vi "PulseGenPan.vi"(8 "error in (no error)":errorcluster caption="entrée d'erreur (pas d'erreur)", 11 "DAQ6363.lvclass":refnum<class "DAQ6363.lvclass">) -> (0 "error out":errorcluster caption="sortie d'erreur", 3 "DAQ6363.lvclass Out":refnum<class "DAQ6363.lvclass">)   [LabVIEW 2019, in "DAQ6363.lvclass"]
uses:
  DAQ6363.lvclass
  C:/Programmes Labview/LabscanV1A/DevicesClass/BaseDevice/BaseDevice.lvclass
  BaseDevice/ClassQueueMess.ctl
  DAQ6363_Func.ctl
  DAQ6363.lvclass/DAQ6363.ctl
  BaseDevice/BaseDevice.lvclass/BaseDevice.ctl
  BaseDevice/Accessor/SetShowInstrNm.vi
  BaseDevice/Accessor/GetClassEvent.vi
  <vilib>/DAQmx/create/channels.llb/DAQmx Create Channel (CI-Count Edges).vi
  <vilib>/DAQmx/create/channels.llb/DAQmx Create Channel (CO-Pulse Generation-Time).vi
  <vilib>/DAQmx/configure/timing.llb/DAQmx Timing (Implicit).vi
  <vilib>/DAQmx/configure/trigger.llb/DAQmx Start Trigger (Digital Edge).vi
  <resource>/objmgr/daqmx.rc
panel:
  in  "MWP":i32=1
  out "APD2GateTask":refnum<k21> caption="tâche en sortie"
  out "Det2CntTask":refnum<k21> caption="tâche en sortie"
  in  "Mw initial delay(s) 2":dbl caption="retard initial" format="%.6f"
  out "LaserLowTime":dbl
  in  "Mw initial delay(s)":dbl caption="retard initial" format="%.6f"
  out "ControlsNames":string[](array[string])
  out "DetCntTask":refnum<k21> caption="tâche en sortie"
  out "APDTask":refnum<k21> caption="tâche en sortie"
  out "MWTask":refnum<k21> caption="tâche en sortie"
  out "LaserTask":refnum<k21> caption="tâche en sortie"
  out "ReadCnts":bool
  in  "DAQ6363 Tabs":enum32{"Main", "Pulsed ODMR", "Advanced"}(tab)
  in  "APD Gate":bool
  in  "Pulse Function":T1(ring)
  in  "Channel 1":bool
  in  "Channel 2":bool
  in  "Rate Graph":bool caption="Rate\nGraph"
  in  "ReadCont":bool caption="Read\nCont."
  out "ReadCounts 2":u32=100 caption="Counts Ch2" min=1 max=100000 step=1
  out "CountsPerSec 2":dbl=100.0 caption="Counts/s Ch2" min=1.0 max=100000.0 step=1.0
  in  "LS_APD_Dl_us 2":dbl=0.02 caption="Laser-APD2\nDelay (us)" min=0.01 max=1000000000.0 step=0.01
  out "ReadCounts":u32=100 caption="Counts Ch1" min=1 max=100000 step=1
  in  "AquireODMR":bool caption="MiseAJour"
  in  "Stop Acq":bool
  in  "APDTime_us":dbl=2.0 caption="APD Gate\nTime (us)" min=0.01 max=1000000000.0 step=0.01
  in  "LS_APD_Dl_us":dbl=0.02 caption="Laser-APD\nDelay (us)" min=0.01 max=1000000000.0 step=0.01
  in  "LS_MW_Dl_us":dbl=0.15 caption="Laser-MW\nDelay (us)" min=0.01 max=1000000000.0 step=0.01
  in  "MW_LS_Dl_us":dbl=0.1 caption="MW-Laser\nDelay (us)" min=0.01 max=1000000000.0 step=0.01
  in  "MWTime_us":dbl=4.0 caption="Microwave\nOn Time (us)" min=0.01 max=1000000000.0 step=0.01
  in  "PulseCount":i32=30000 caption="Avg. Pulses" min=1 step=1
  in  "LaserTime_us":dbl=10.0 caption="Laser On\nTime (us)" min=0.01 max=1000000000.0 step=0.01
  out "AcqTime":dbl caption="AcqTime(s)" format="%<%M:%S%3u>t"
  out "CountsPerSec":dbl=100.0 caption="Counts/s Ch1" min=1.0 max=100000.0 step=1.0
  out "Period(us)":dbl
  in  "DetInput2":tag="/Dev1/PFI8" caption="Detection Input 2"
  in  "DetCntr 2":tag="Dev1/ctr3" caption="Detection Counter 2"
  in  "APDOutput 2":tag="/Dev1/PFI11" caption="APD Gate In/Out 2"
  in  "APDGateCntr2":tag="Dev1/ctr2" caption="APD Gate Counter 2"
  in  "DetInput":tag="/Dev1/PFI13" caption="Detection Input"
  in  "DetCntr":tag="Dev1/ctr0" caption="Detection Counter"
  in  "APDCntr":tag="Dev1/ctr1" caption="APD Gate Counter"
  in  "APDOutput":tag="/Dev1/PFI10" caption="APD Gate In/Out"
  in  "MWCntr":tag="Dev1/ctr2" caption="Microwave Counter"
  in  "LaserCntr":tag="Dev1/ctr1" caption="Laser Counter"
  in  "Laser In/Out":tag="/Dev1/PFI9" caption="LaserTrig In/Out"
  in  "MW In/Out":tag="/Dev1/PFI12" caption="Microwave In/Out"
  in  "APDGateEdge":i32(ring)=10280 items=["Montant"=10280, "Descendant"=10171]
  in  "MainProgQ":refnum<queue>
  in  "MainProgQEvent":refnum<user-event>
  in  "Acq":bool
  in  "Stop":bool
  out "Init Program":bool
  # "DAQ6363 Pulse Gen"
  # "this MUST labeled with class name"
  # "this MUST be present and labeled \"Stop\" and \"Acq\""
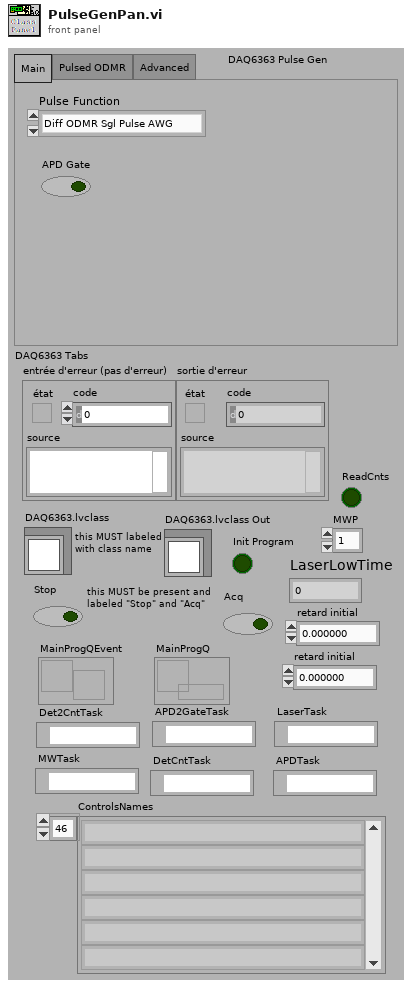
[diagram p1: front panel]
types:
  T1 = enum16{"Diff ODMR Sgl Pulse AWG", "Pulsed ODMR AWG", "Diff Pulsed ODMR AWG", "Pulsed ODMR", "Diff Pulsed ODMR", "Ramsey", "Rabi", "Gated Pulse Count", "None"}
  T2 = typedef "DAQ6363.lvclass/DAQ6363_Func.ctl" = enum16{"CountPulse (Cnt)", "Rabi (Tau)", "MWtoLaserDelay (us)", "APDGate (us)", "PulsedODMR (Pulses)", "PulsedODMR_AWG (Pulses)", "DiffODMRSglPulseAWG (Pulses)", "DiffPulsedODMR_AWG (Pulses)", "GatedPulseCount (Pulses)", "DiffPulsedODMR (Pulses)"}
  T3 = typedef "ClassQueueMess.ctl" = u16
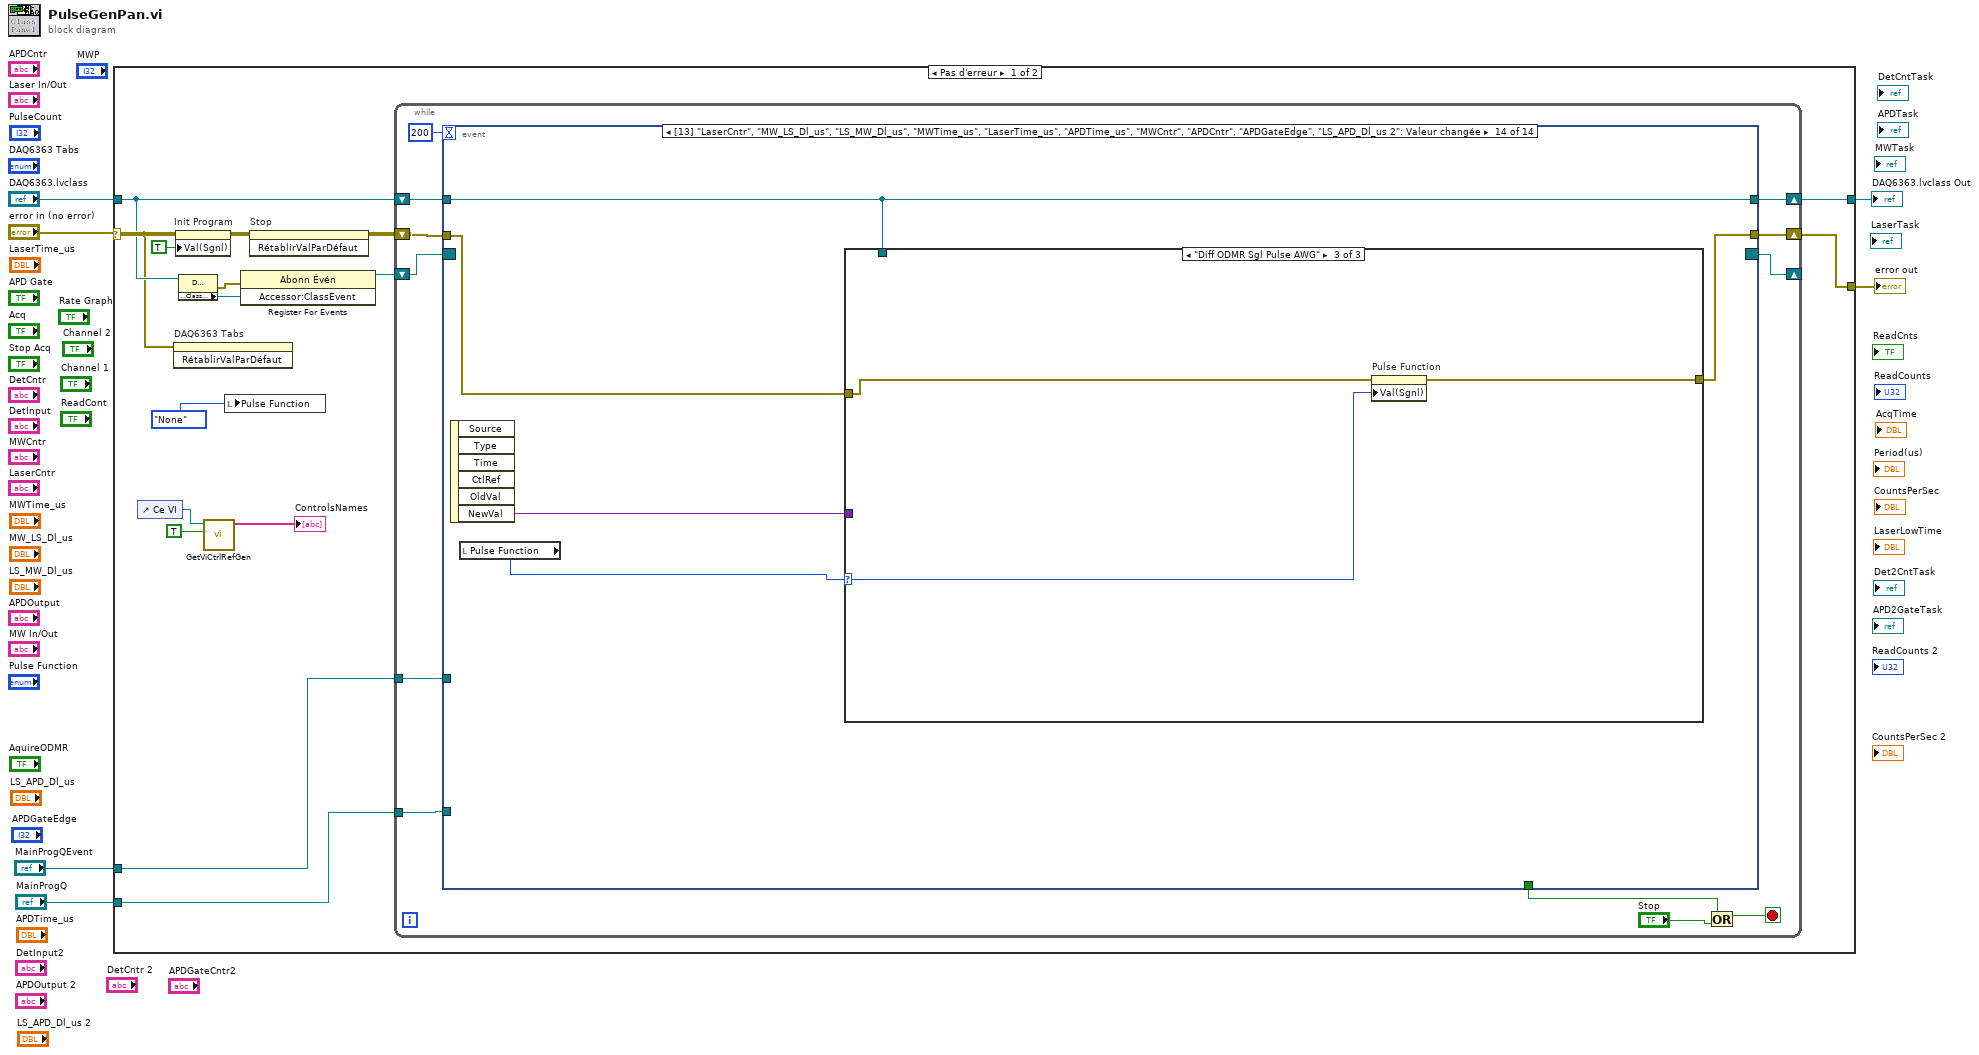
[diagram p0: block diagram]
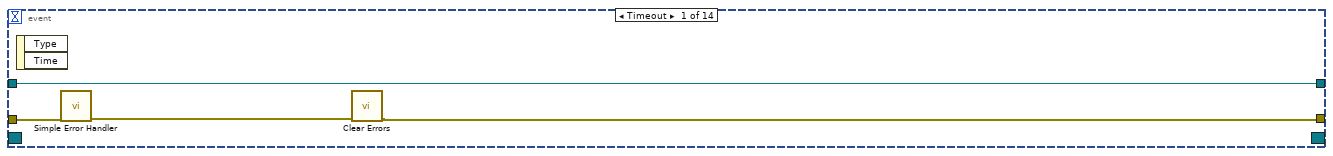
[diagram p2: hidden frame]
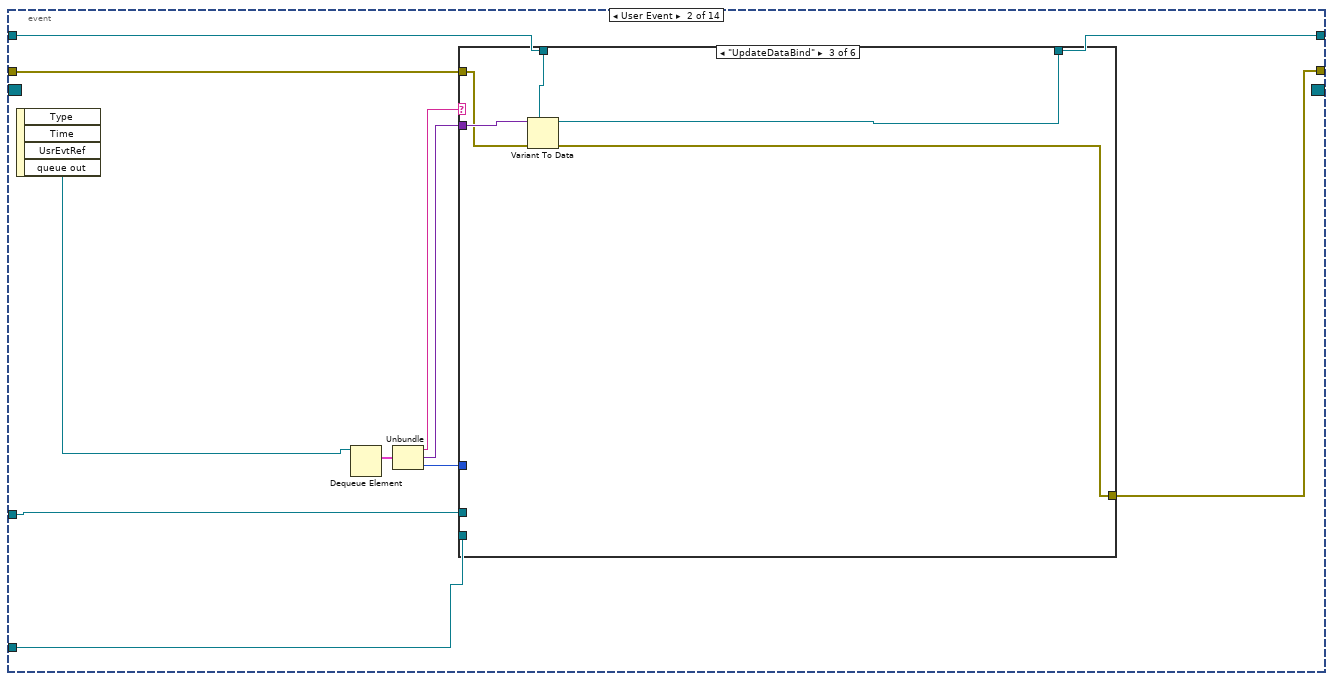
[diagram p3: hidden frame]
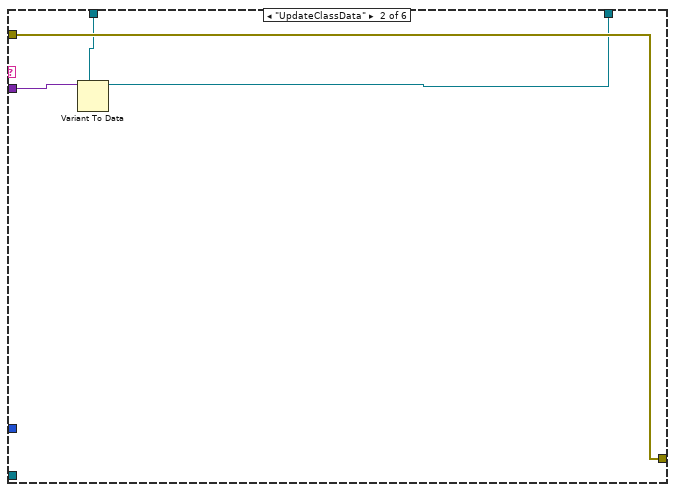
[diagram p5: hidden frame]
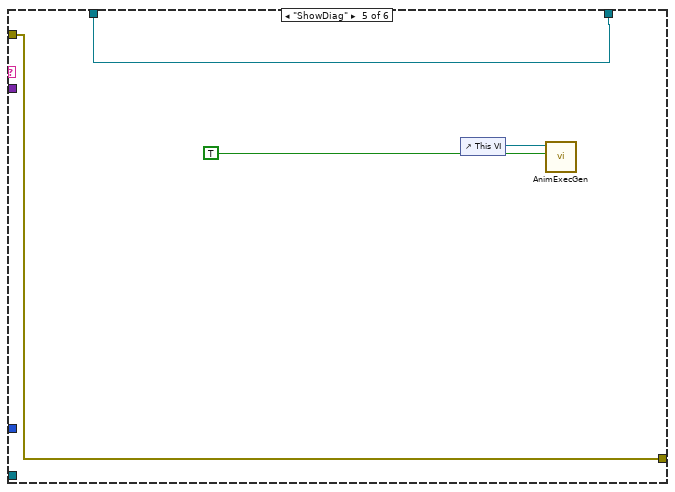
[diagram p7: hidden frame]
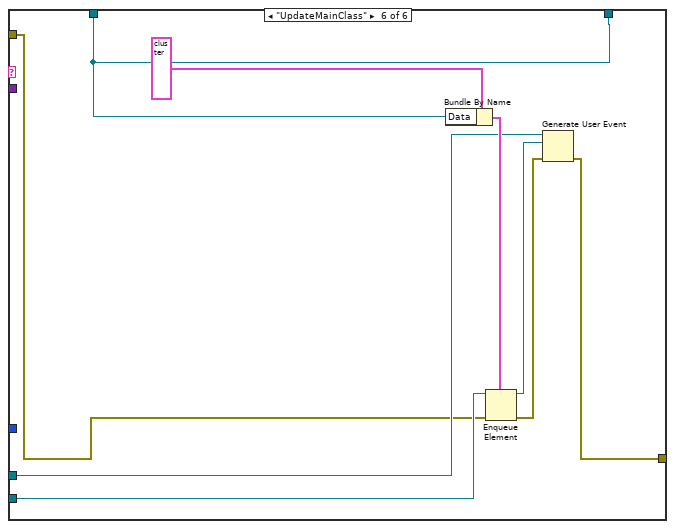
[diagram p8: hidden frame]
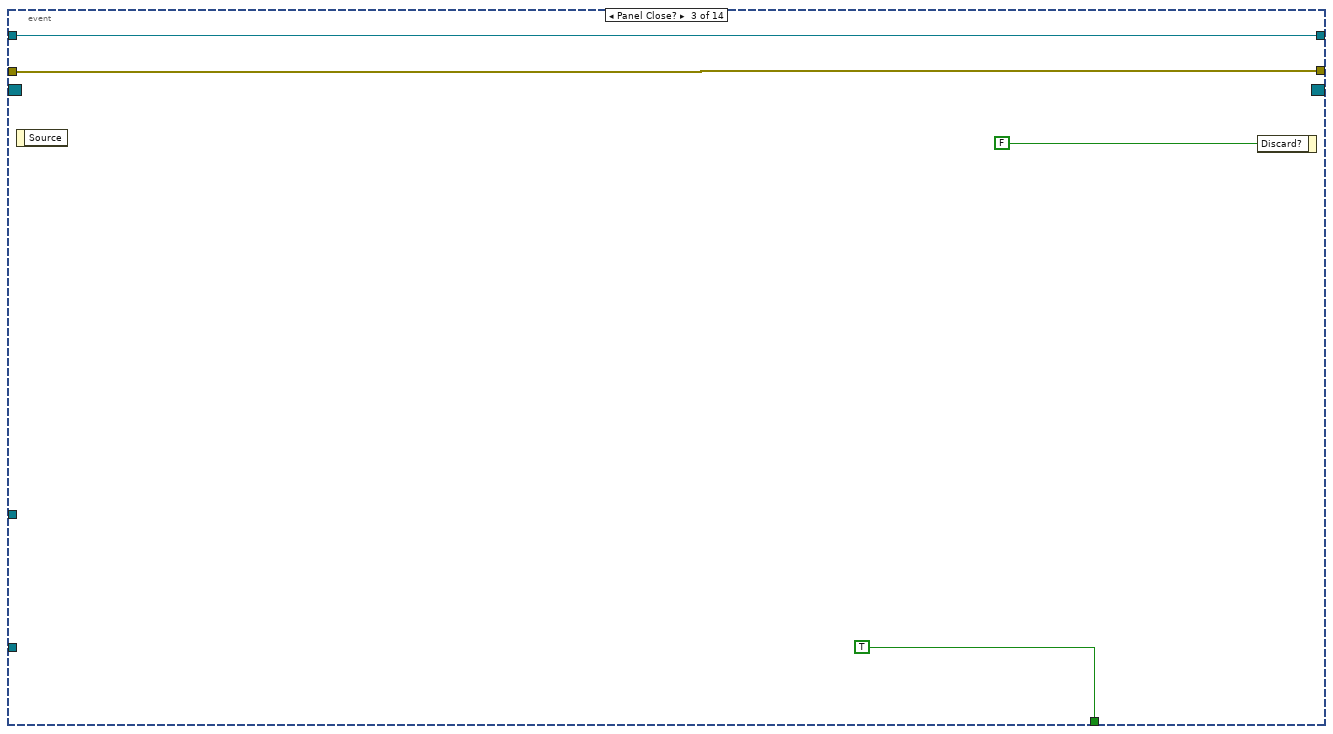
[diagram p9: hidden frame]
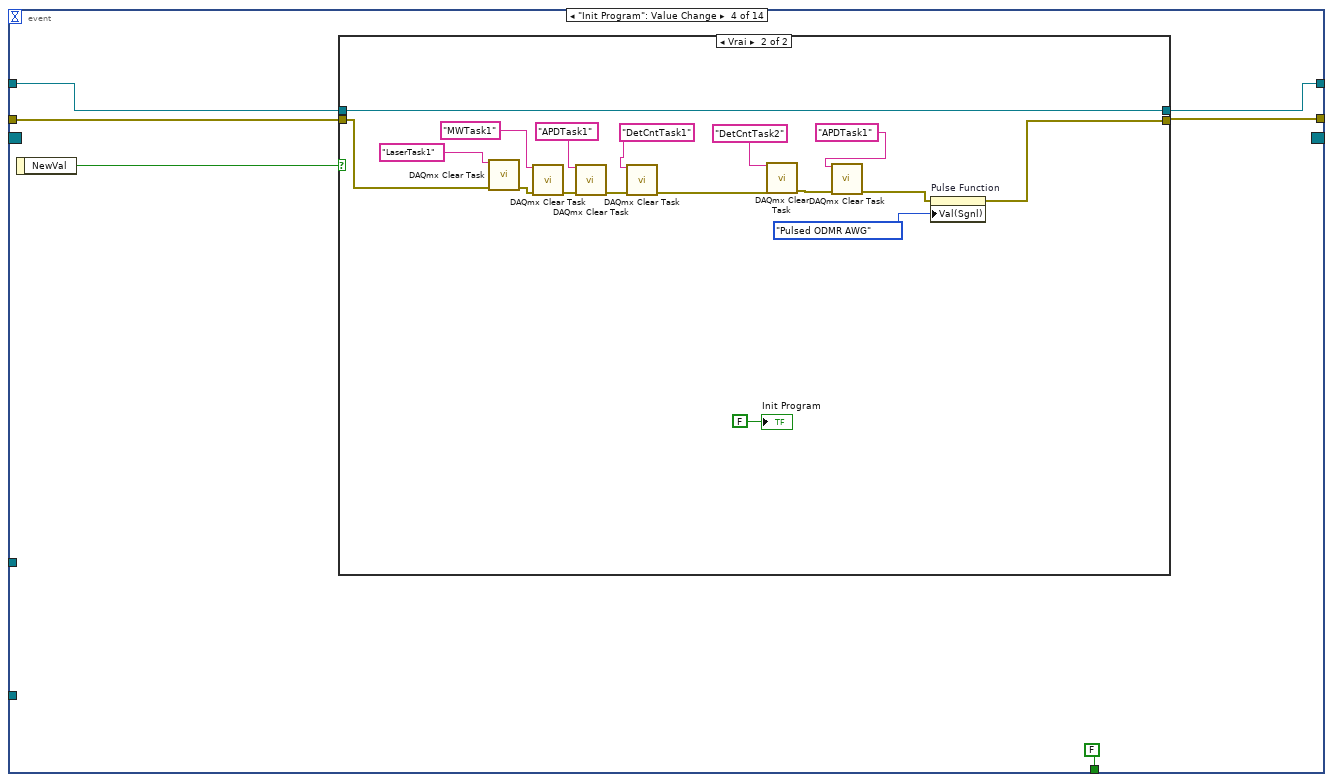
[diagram p10: hidden frame]
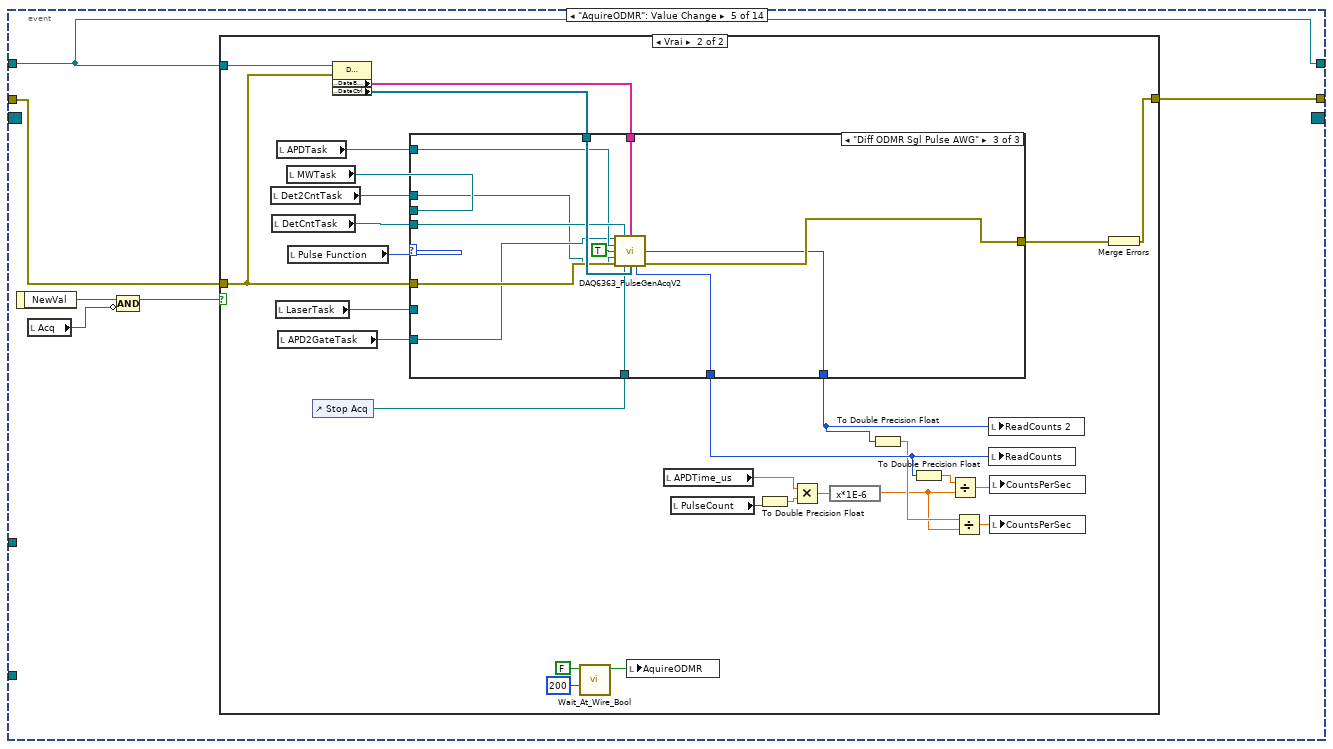
[diagram p12: hidden frame]
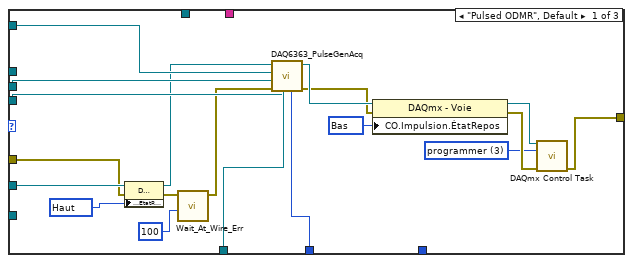
[diagram p14: hidden frame]
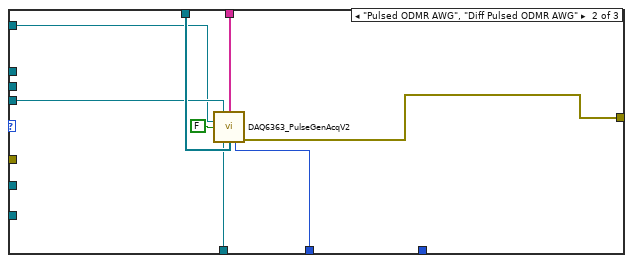
[diagram p15: hidden frame]
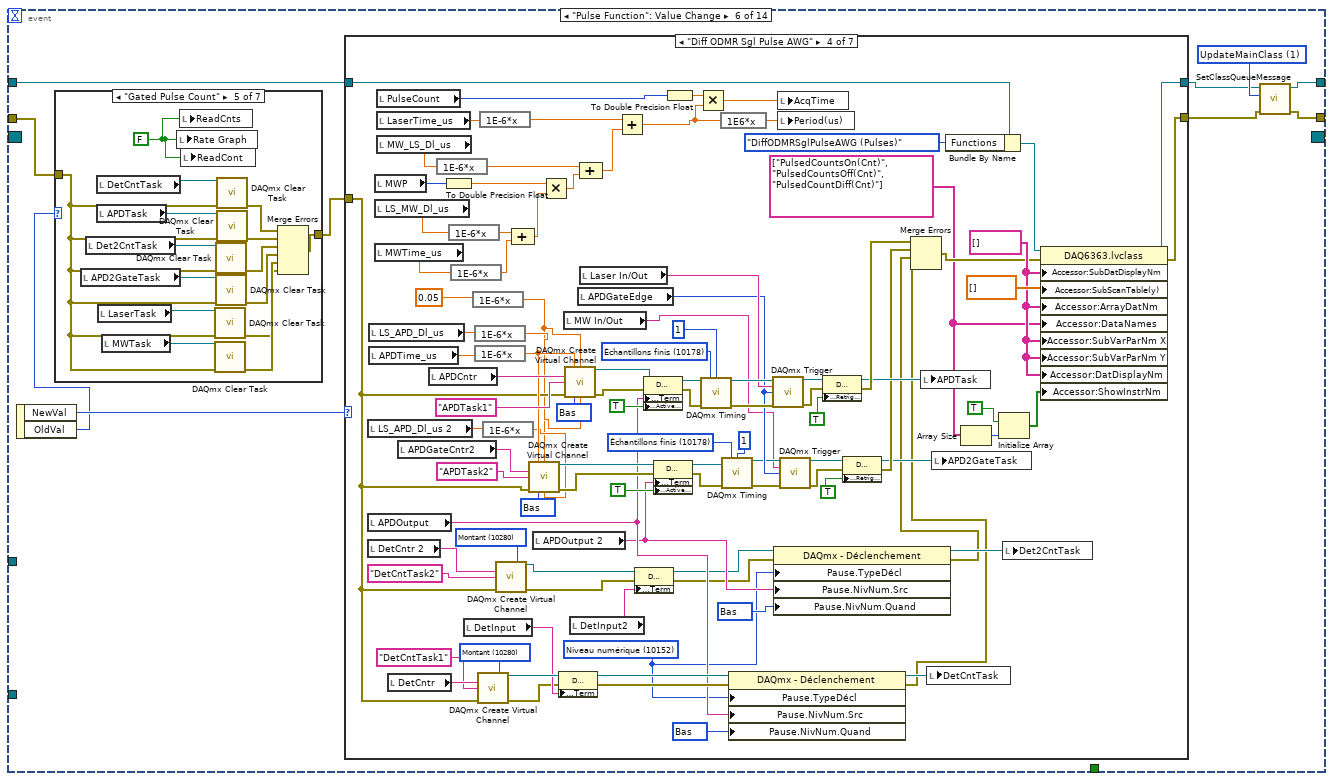
[diagram p16: hidden frame]
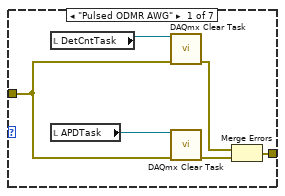
[diagram p17: hidden frame]
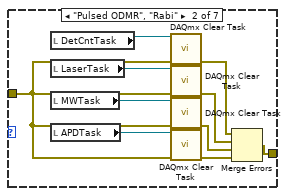
[diagram p18: hidden frame]
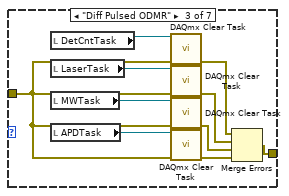
[diagram p19: hidden frame]
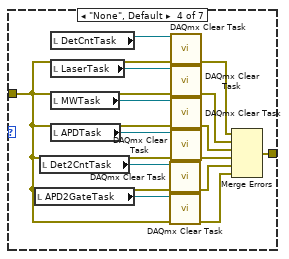
[diagram p20: hidden frame]
diagram:
  n1 = case shown="Pas d'erreur" "error in (no error)" {
    selector: "error in (no error)" -> [w11 w908]
    tunnel: [w22 w908] -> w5
    tunnel: "DAQ6363.lvclass" -> [w15 w907]
    tunnel: [w20 w907] -> w3
    tunnel: "MainProgQEvent" -> [w13 _]
    tunnel: "MainProgQ" -> [w12 _]
    frame No Error {
      n2 = control-ref of="Ce VI"() -> (w9:refnum<vi>)
      n3 = invoke on="DAQ6363 Tabs" class="Onglet (strict)" method="RétablirValParDéfaut"(error in=w11) -> ()  [unwired: 2 in, 3 out]
      n4 = property on="Init Program" class="Bool (strict)"(error in=w11, "Val(Sgnl)"=TRUE ("Valeur (Signalisation)")) -> (error out=w19:errorcluster)  [unwired: 1 in, 1 out]
      n5 = property class="DAQ6363.lvclass"(reference=w15) -> (error out=w17:errorcluster, "Accessor:ClassEvent"=w16:refnum<user-event>)  [unwired: 1 in, 1 out]
      n6 = call <userlib>:"GetViCtrlRefGen.vi"("InclTabCTrl"=TRUE, "VIRef"=w9) -> ("ControlsNames"=→"ControlsNames":string[])  [unwired: 7 in, 2 out]
      n7 = local write "Pulse Function"(T1."None" ("Pulse Function")) -> ()
      n8 = register-events(error in=w17, w16) -> (reference out=w14:refnum<event-registration>)  [unwired: 1 in, 1 out]
      n9 = invoke on="Stop" class="Bool (strict)" method="RétablirValParDéfaut"(error in=w19) -> (error out=w18:errorcluster)  [unwired: 2 in, 2 out]
      n10 = while {
        shift-right: [w32] -> w22
        shift-left: w18 -> [w33]
        shift-right: [w30] -> w20
        shift-left: w15 -> [w31]
        shift-right: [w26] -> _
        shift-left: w14 -> [w27]
        tunnel: w13 -> [w25]
        tunnel: w12 -> [w24]
        stop <- w29 stop-if-true
        n11 = event shown="[13] \"LaserCntr\", \"MW_LS_Dl_us\", \"LS_MW_Dl_us\", \"MWTime_us\", \"LaserTime_us\", \"APDTime_us\", \"MWCntr\", \"APDCntr\", \"APDGateEdge\", \"LS_APD_Dl_us 2\": Valeur changée" {
          selector: w27 -> [_ _ _ _ _ _ _ _ _ _ _ _ _ _]
          dyn-events: [_ _ _ _ _ _ _ _ _ _ _ _ _ _] -> w26
          timeout: 200 -> [_ _ _ _ _ _ _ _ _ _ _ _ _ _]
          tunnel: w33 -> [w38 w48 w77 w84 w109 w180 w722 w781 w827 w843 w867 w877 w887 w897]
          tunnel: [w35 w42 w77 w83 w108 w186 w719 w778 w829 w842 w866 w876 w886 w896] -> w32
          tunnel: w31 -> [w36 w49 w76 w81 w105 w188 w723 w782 w830 w844 w868 w878 w888 w898]
          tunnel: [w36 w41 w76 w80 w105 w184 w717 w776 w830 w844 w868 w878 w888 w898] -> w30
          tunnel: w25 -> [_ w40 _ _ _ _ _ _ _ _ _ _ _ _]
          tunnel: w24 -> [_ w39 _ _ _ _ _ _ _ _ _ _ _ _]
          tunnel: [_ _ TRUE FALSE _ _ _ _ _ _ _ _ _ _] -> w23
          event Timeout {
            n12 = event-data() -> ()  [unwired: 1 in, 2 out]
            n13 = call <vilib>:"Simple Error Handler.vi"("error in (no error)"=w38) -> ("error out"=w37:errorcluster)  [unwired: 4 in, 4 out]
            n14 = call <vilib>:"Clear Errors.vi"("error in (no error)"=w37) -> ("error out"=w35:errorcluster)  [unwired: 5 in, 1 out]
          }
          event User Event {
            n15 = event-data() -> ("queue out"=w46:refnum<queue>)  [unwired: 1 in, 3 out]
            n16 = Dequeue Element(queue=w46) -> (element=w47:cluster{"Message":string, "Data":variant, i32})  [unwired: 2 in, 3 out]
            n17 = Unbundle(w47) -> ("Message"=w45:string, "Data"=w44:variant, w43:i32)
            n18 = case shown="\"UpdateDataBind\"" w45 {
              tunnel: w48 -> [w51 w55 w57 w61 w65 w68]
              tunnel: w44 -> [_ w54 w60 _ _ _]
              tunnel: w49 -> [w50 w53 w59 w62 w66 w71]
              tunnel: [w50 w52 w58 w62 w66 w71] -> w41
              tunnel: [w51 w55 w56 w61 w65 w67] -> w42
              tunnel: w43 -> [_ _ _ _ _ _]
              tunnel: w40 -> [_ _ _ _ _ w70]
              tunnel: w39 -> [_ _ _ _ _ w69]
              frame Default {
              }
              frame "UpdateClassData" {
                n19 = Variant To Data(type=w53, Variant=w54) -> (data=w52:refnum<class "DAQ6363.lvclass">)  [unwired: 1 in, 1 out]
              }
              frame "UpdateDataBind" {
                n20 = Variant To Data(error in=w57, type=w59, Variant=w60) -> (data=w58:refnum<class "DAQ6363.lvclass">, error out=w56:errorcluster)
              }
              frame "MeasDone" {
              }
              frame "ShowDiag" {
                n21 = control-ref of="This VI"() -> (w64:refnum<vi>)
                n22 = call <userlib>:"AnimExecGen.vi"("Animer l'exécution ?"=TRUE, "ViRef"=w64) -> ()  [unwired: 9 in, 1 out]
              }
              frame "UpdateMainClass" {
                n23 = Bundle By Name(cluster=cluster{"Message":string, "Data":variant, i32} {"Message"="", "Data"=variant, 0} ("élément"), "Data"=w71) -> (w72:cluster{"Message":string, "Data":variant, i32})
                n24 = Enqueue Element(queue=w69, element=w72, error in (no error)=w68) -> (queue out=w75:refnum<queue>, error out=w74:errorcluster)  [unwired: 1 in, 1 out]
                n25 = Generate User Event(user event=w70, event data cluster=w75, error in=w74) -> (error out=w67:errorcluster)  [unwired: 1 in, 1 out]
              }
            }
          }
          event Panel Close? {
            n26 = event-data() -> ()  [unwired: 1 in, 1 out]
            n27 = event-data("Discard?"=FALSE ("Rejeter ?")) -> ()  [unwired: 1 in, 1 out]
          }
          event "Init Program": Value Change {
            n28 = event-data() -> ("NewVal"=w85:bool)  [unwired: 1 in]
            n29 = case shown="Vrai" w85 {
              tunnel: w84 -> [w87 w101]
              tunnel: [w87 w89] -> w83
              tunnel: [w86 w103] -> w80
              tunnel: w81 -> [w86 w103]
              frame False {
              }
              frame True {
                n30 = call <vilib>:"DAQmx Clear Task.vi"("task in"="LaserTask1" ("name to assign"), "error in"=w101) -> ("error out"=w98:errorcluster)  [unwired: 13 in]
                n31 = call <vilib>:"DAQmx Clear Task.vi"("task in"="MWTask1" ("name to assign"), "error in"=w98) -> ("error out"=w97:errorcluster)  [unwired: 13 in]
                n32 = call <vilib>:"DAQmx Clear Task.vi"("task in"="APDTask1" ("name to assign"), "error in"=w97) -> ("error out"=w95:errorcluster)  [unwired: 13 in]
                n33 = call <vilib>:"DAQmx Clear Task.vi"("task in"="DetCntTask1" ("name to assign"), "error in"=w95) -> ("error out"=w93:errorcluster)  [unwired: 13 in]
                n34 = call <vilib>:"DAQmx Clear Task.vi"("task in"="DetCntTask2" ("name to assign"), "error in"=w93) -> ("error out"=w94:errorcluster)  [unwired: 13 in]
                n35 = call <vilib>:"DAQmx Clear Task.vi"("task in"="APDTask1" ("name to assign"), "error in"=w94) -> ("error out"=w90:errorcluster)  [unwired: 13 in]
                n36 = property on="Pulse Function" class="Énum (strict)"(error in=w90, "Val(Sgnl)"=T1."Pulsed ODMR AWG" ("Valeur (Signalisation)")) -> (error out=w89:errorcluster)  [unwired: 1 in, 1 out]
                "Init Program" <- FALSE
              }
            }
          }
          event "AquireODMR": Value Change {
            n37 = event-data() -> ("NewVal"=w110:bool)  [unwired: 1 in]
            n38 = local read "Acq"() -> (w106:bool)
            n39 = Compound Arithmetic op=AND ("Opérateur arithmétique")(w110, invert w106) -> (w107:bool)
            n40 = case shown="Vrai" w107 {
              tunnel: w109 -> [w111 w112]
              tunnel: [w111 w136] -> w108
              tunnel: w105 -> [_ w123]
              frame False {
              }
              frame True {
                n41 = local read "Det2CntTask"() -> (w118:refnum<k21>)
                n42 = local read "DetCntTask"() -> (w124:refnum<k21>)
                n43 = local read "LaserTask"() -> (w120:refnum<k21>)
                n44 = local read "APDTask"() -> (w127:refnum<k21>)
                n45 = local read "APD2GateTask"() -> (w117:refnum<k21>)
                n46 = local read "MWTask"() -> (w126:refnum<k21>)
                n47 = local read "Pulse Function"() -> (w125:T1)
                n48 = control-ref of="Stop Acq"() -> (w128:refnum<vi>)
                n49 = property class="DAQ6363.lvclass"(reference=w123, error in=w112) -> ("Accessor:DataBindCtrl"=w122:string[], "Accessor:DataCtrl"=w121:refnum<vi>[])  [unwired: 2 out]
                n50 = case shown="\"Diff ODMR Sgl Pulse AWG\"" w125 {
                  tunnel: [w147 w160 w172] -> w129
                  tunnel: w128 -> [w158 w163 w175]
                  tunnel: w127 -> [w157 w161 w173]
                  tunnel: w126 -> [w156 _ _]
                  tunnel: w124 -> [w155 w162 w174]
                  tunnel: w122 -> [_ w165 w177]
                  tunnel: w121 -> [_ w164 w176]
                  tunnel: w120 -> [w152 _ _]
                  tunnel: w112 -> [w151 _ w170]
                  tunnel: [w140 w159 w171] -> w119
                  tunnel: w118 -> [_ _ w168]
                  tunnel: w117 -> [_ _ w169]
                  tunnel: [_ _ w167] -> w116
                  frame "Pulsed ODMR", Default {
                    w144 = 3 items=["vérifier"=2, "réserver"=4, "programmer"=3, "libérer"=5, "abandonner"=6] ("action")
                    w141 = 10214 items=["Haut"=10192, "Bas"=10214] ("CO.Impulsion.ÉtatRepos")
                    w150 = 10192 items=["Haut"=10192, "Bas"=10214] ("CO.Impulsion.ÉtatRepos")
                    n51 = property class="DAQmx - Voie"(reference=w152, error in=w151, "CO.Impulsion.ÉtatRepos"=w150) -> (reference out=w148:refnum<k21>, error out=w154:errorcluster)
                    n52 = call <userlib>:"Wait_At_Wire_Err.vi"("Wait (ms)"=u32 100, "error in (no error)"=w154) -> ("error out"=w149:errorcluster)  [unwired: 7 in, 2 out]
                    n53 = call <userlib>:"DAQ6363_PulseGenAcq.vi"("HaltRef"=w158, "CntTaskIn"=w155, "error in (no error)"=w149, "MWTaskIn"=w156, "APDTaskIn"=w157, "LaserTaskIn"=w148) -> ("error out"=w142:errorcluster, "LaserTaskOut"=w143:refnum<k21>, "Counts Out"=w147:u32)  [unwired: 3 out]
                    n54 = property class="DAQmx - Voie"(reference=w143, error in=w142, "CO.Impulsion.ÉtatRepos"=w141) -> (reference out=w145:refnum<k21>, error out=w146:errorcluster)
                    n55 = call <vilib>:"DAQmx Control Task.vi"("task/channels in"=w145, "action"=w144, "error in"=w146) -> ("error out"=w140:errorcluster)  [unwired: 11 in, 1 out]
                  }
                  frame "Pulsed ODMR AWG", "Diff Pulsed ODMR AWG" {
                    n56 = call <userlib>:"DAQ6363_PulseGenAcqV2.vi"("A1CntTaskIn"=w162, "DataBindCtrlNm"=w165, "APD1GTaskIn"=w161, "APD2_On"=FALSE, "HaltRef"=w163, "Control Ref"=w164) -> ("A1Counts Out"=w160:u32, "error out"=w159:errorcluster)  [unwired: 3 in, 5 out]
                  }
                  frame "Diff ODMR Sgl Pulse AWG" {
                    n57 = call <userlib>:"DAQ6363_PulseGenAcqV2.vi"("APD2GTaskIn"=w169, "A1CntTaskIn"=w174, "DataBindCtrlNm"=w177, "APD1GTaskIn"=w173, "APD2_On"=TRUE, "A2CntTaskIn"=w168, "error in (no error)"=w170, "HaltRef"=w175, "Control Ref"=w176) -> ("A2Counts Out"=w167:u32, "A1Counts Out"=w172:u32, "error out"=w171:errorcluster)  [unwired: 4 out]
                  }
                }
                n58 = call <userlib>:"Wait_At_Wire_Bool.vi"("Wait (ms)"=u32 200, "error in (no error)"=FALSE) -> ("error out"=w139:bool)  [unwired: 7 in, 2 out]
                n59 = local write "AquireODMR"(w139) -> ()
                n60 = local read "APDTime_us"() -> (w135:dbl)
                n61 = local read "PulseCount"() -> (w134:i32)
                n62 = To Double Precision Float(number=w134) -> (double precision float=w133:dbl)
                n63 = Multiply(x=w135, y=w133) -> (x*y=w132:dbl)
                n64 = expression code="x*1E-6"(w132) -> (w114:dbl)
                n65 = To Double Precision Float(number=w116) -> (double precision float=w115:dbl)
                n66 = To Double Precision Float(number=w129) -> (double precision float=w131:dbl)
                n67 = Divide(x=w131, y=w114) -> (x/y=w130:dbl)
                n68 = Divide(x=w115, y=w114) -> (x/y=w113:dbl)
                n69 = local write "ReadCounts 2"(w116) -> ()
                n70 = local write "ReadCounts"(w129) -> ()
                n71 = local write "CountsPerSec"(w130) -> ()
                n72 = local write "CountsPerSec"(w113) -> ()
                n73 = Merge Errors(w119) -> (w136:errorcluster)
              }
            }
          }
          event "Pulse Function": Value Change {
            w187 = T3 1 items=["UpdateClassData", "UpdateMainClass", "UpdateDataBind", "ReInitDevice", "Custom", "ClosePan"] ("Menu déroulant")
            n74 = event-data() -> ("NewVal"=w183:T1, "OldVal"=w181:T1)  [unwired: 1 in]
            n75 = case shown="\"Gated Pulse Count\"" w181 {
              tunnel: [w191 w198 w208 w222 w240 w248 w254] -> w182
              tunnel: w180 -> [w190 w195 w205 w217 w232 w245 w253]
              frame "Pulsed ODMR AWG" {
                n76 = local read "DetCntTask"() -> (w193:refnum<k21>)
                n77 = local read "APDTask"() -> (w194:refnum<k21>)
                n78 = call <vilib>:"DAQmx Clear Task.vi"("task in"=w193, "error in"=w190) -> ("error out"=w189:errorcluster)  [unwired: 13 in]
                n79 = call <vilib>:"DAQmx Clear Task.vi"("task in"=w194, "error in"=w190) -> ("error out"=w192:errorcluster)  [unwired: 13 in]
                n80 = Merge Errors(w189, w192) -> (w191:errorcluster)
              }
              frame "Pulsed ODMR", "Rabi" {
                n81 = local read "DetCntTask"() -> (w201:refnum<k21>)
                n82 = local read "LaserTask"() -> (w202:refnum<k21>)
                n83 = local read "MWTask"() -> (w203:refnum<k21>)
                n84 = local read "APDTask"() -> (w204:refnum<k21>)
                n85 = call <vilib>:"DAQmx Clear Task.vi"("task in"=w201, "error in"=w195) -> ("error out"=w199:errorcluster)  [unwired: 13 in]
                n86 = call <vilib>:"DAQmx Clear Task.vi"("task in"=w202, "error in"=w195) -> ("error out"=w197:errorcluster)  [unwired: 13 in]
                n87 = call <vilib>:"DAQmx Clear Task.vi"("task in"=w203, "error in"=w195) -> ("error out"=w196:errorcluster)  [unwired: 13 in]
                n88 = call <vilib>:"DAQmx Clear Task.vi"("task in"=w204, "error in"=w195) -> ("error out"=w200:errorcluster)  [unwired: 13 in]
                n89 = Merge Errors(w199, w197, w196, w200) -> (w198:errorcluster)
              }
              frame "Diff Pulsed ODMR" {
                n90 = local read "DetCntTask"() -> (w211:refnum<k21>)
                n91 = local read "LaserTask"() -> (w212:refnum<k21>)
                n92 = local read "MWTask"() -> (w213:refnum<k21>)
                n93 = local read "APDTask"() -> (w214:refnum<k21>)
                n94 = call <vilib>:"DAQmx Clear Task.vi"("task in"=w211, "error in"=w205) -> ("error out"=w209:errorcluster)  [unwired: 13 in]
                n95 = call <vilib>:"DAQmx Clear Task.vi"("task in"=w212, "error in"=w205) -> ("error out"=w207:errorcluster)  [unwired: 13 in]
                n96 = call <vilib>:"DAQmx Clear Task.vi"("task in"=w213, "error in"=w205) -> ("error out"=w206:errorcluster)  [unwired: 13 in]
                n97 = call <vilib>:"DAQmx Clear Task.vi"("task in"=w214, "error in"=w205) -> ("error out"=w210:errorcluster)  [unwired: 13 in]
                n98 = Merge Errors(w209, w207, w206, w210) -> (w208:errorcluster)
              }
              frame "None", Default {
                n99 = local read "APD2GateTask"() -> (w218:refnum<k21>)
                n100 = local read "Det2CntTask"() -> (w219:refnum<k21>)
                n101 = local read "DetCntTask"() -> (w225:refnum<k21>)
                n102 = local read "LaserTask"() -> (w226:refnum<k21>)
                n103 = local read "MWTask"() -> (w227:refnum<k21>)
                n104 = local read "APDTask"() -> (w228:refnum<k21>)
                n105 = call <vilib>:"DAQmx Clear Task.vi"("task in"=w219, "error in"=w217) -> ("error out"=w216:errorcluster)  [unwired: 13 in]
                n106 = call <vilib>:"DAQmx Clear Task.vi"("task in"=w218, "error in"=w217) -> ("error out"=w215:errorcluster)  [unwired: 13 in]
                n107 = call <vilib>:"DAQmx Clear Task.vi"("task in"=w225, "error in"=w217) -> ("error out"=w223:errorcluster)  [unwired: 13 in]
                n108 = call <vilib>:"DAQmx Clear Task.vi"("task in"=w226, "error in"=w217) -> ("error out"=w221:errorcluster)  [unwired: 13 in]
                n109 = call <vilib>:"DAQmx Clear Task.vi"("task in"=w227, "error in"=w217) -> ("error out"=w220:errorcluster)  [unwired: 13 in]
                n110 = call <vilib>:"DAQmx Clear Task.vi"("task in"=w228, "error in"=w217) -> ("error out"=w224:errorcluster)  [unwired: 13 in]
                n111 = Merge Errors(w223, w221, w220, w224, w216, w215) -> (w222:errorcluster)
              }
              frame "Gated Pulse Count" {
                w236 = FALSE ("Rate Graph")
                n112 = local read "APD2GateTask"() -> (w238:refnum<k21>)
                n113 = local read "Det2CntTask"() -> (w239:refnum<k21>)
                n114 = local read "DetCntTask"() -> (w242:refnum<k21>)
                n115 = local read "APDTask"() -> (w243:refnum<k21>)
                n116 = local read "LaserTask"() -> (w233:refnum<k21>)
                n117 = local read "MWTask"() -> (w231:refnum<k21>)
                n118 = local write "Rate Graph"(w236) -> ()
                n119 = local write "ReadCnts"(w236) -> ()
                n120 = local write "ReadCont"(w236) -> ()
                n121 = call <vilib>:"DAQmx Clear Task.vi"("task in"=w233, "error in"=w232) -> ("error out"=w229:errorcluster)  [unwired: 13 in]
                n122 = call <vilib>:"DAQmx Clear Task.vi"("task in"=w231, "error in"=w232) -> ("error out"=w230:errorcluster)  [unwired: 13 in]
                n123 = call <vilib>:"DAQmx Clear Task.vi"("task in"=w239, "error in"=w232) -> ("error out"=w234:errorcluster)  [unwired: 13 in]
                n124 = call <vilib>:"DAQmx Clear Task.vi"("task in"=w238, "error in"=w232) -> ("error out"=w235:errorcluster)  [unwired: 13 in]
                n125 = call <vilib>:"DAQmx Clear Task.vi"("task in"=w242, "error in"=w232) -> ("error out"=w237:errorcluster)  [unwired: 13 in]
                n126 = call <vilib>:"DAQmx Clear Task.vi"("task in"=w243, "error in"=w232) -> ("error out"=w241:errorcluster)  [unwired: 13 in]
                n127 = Merge Errors(w237, w241, w234, w235, w230, w229) -> (w240:errorcluster)
              }
              frame "Diff ODMR Sgl Pulse AWG" {
                n128 = local read "APD2GateTask"() -> (w246:refnum<k21>)
                n129 = local read "Det2CntTask"() -> (w247:refnum<k21>)
                n130 = local read "DetCntTask"() -> (w250:refnum<k21>)
                n131 = local read "APDTask"() -> (w251:refnum<k21>)
                n132 = call <vilib>:"DAQmx Clear Task.vi"("task in"=w247, "error in"=w245) -> ()  [unwired: 13 in, 1 out]
                n133 = call <vilib>:"DAQmx Clear Task.vi"("task in"=w246, "error in"=w245) -> ()  [unwired: 13 in, 1 out]
                n134 = call <vilib>:"DAQmx Clear Task.vi"("task in"=w250, "error in"=w245) -> ("error out"=w244:errorcluster)  [unwired: 13 in]
                n135 = call <vilib>:"DAQmx Clear Task.vi"("task in"=w251, "error in"=w245) -> ("error out"=w249:errorcluster)  [unwired: 13 in]
                n136 = Merge Errors(w244, w249) -> (w248:errorcluster)
              }
              frame "Diff Pulsed ODMR AWG" {
                n137 = local read "DetCntTask"() -> (w256:refnum<k21>)
                n138 = local read "APDTask"() -> (w257:refnum<k21>)
                n139 = call <vilib>:"DAQmx Clear Task.vi"("task in"=w256, "error in"=w253) -> ("error out"=w255:errorcluster)  [unwired: 13 in]
                n140 = call <vilib>:"DAQmx Clear Task.vi"("task in"=w257, "error in"=w253) -> ("error out"=w252:errorcluster)  [unwired: 13 in]
                n141 = Merge Errors(w255, w252) -> (w254:errorcluster)
              }
            }
            n142 = case shown="\"Diff ODMR Sgl Pulse AWG\"" w183 {
              tunnel: [w314 w399 w467 w569 w597 w669 w708] -> w185
              tunnel: w188 -> [w260 w361 w429 w535 w594 w614 w708]
              tunnel: w182 -> [w308 w360 w428 w504 w592 w663 w707]
              tunnel: [w315 w400 w468 w570 w598 w670 w707] -> w179
              frame "Pulsed ODMR", "Rabi" {
                w276 = 10214 items=["Haut"=10192, "Bas"=10214] ("Pause.NivNum.Quand")
                w280 = 10152 items=["Niveau analogique"=10101, "Fenêtre analogique"=10103, "Niveau numérique"=10152, "Pattern numérique"=10398, "Aucun"=10230] ("Pause.TypeDécl")
                w289 = 10171 items=["Montant"=10280, "Descendant"=10171] ("edge")
                w310 = 10280 items=["Montant"=10280, "Descendant"=10171] ("edge")
                w320 = string[] [] ("SubDatDisplayNm")
                w316 = string[] ["PulsedCounts(Cnt)"]
                w323 = 10178 items=["Échantillons finis"=10178, "Échantillons continus"=10123, "Point par point avec cadencement matériel"=12522] ("sample mode")
                w332 = 10214 items=["Haut"=10192, "Bas"=10214] ("idle state")
                w334 = 10214 items=["Haut"=10192, "Bas"=10214] ("idle state")
                w336 = 10178 items=["Échantillons finis"=10178, "Échantillons continus"=10123, "Point par point avec cadencement matériel"=12522] ("sample mode")
                w347 = 10192 items=["Haut"=10192, "Bas"=10214] ("idle state")
                w352 = 10178 items=["Échantillons finis"=10178, "Échantillons continus"=10123, "Point par point avec cadencement matériel"=12522]  # Mode d'échantillonnage
                n143 = local read "LS_MW_Dl_us"() -> (w298:dbl)
                n144 = local read "MWTime_us"() -> (w296:dbl)
                n145 = local read "MW_LS_Dl_us"() -> (w294:dbl)
                n146 = local read "MWP"() -> (w263:i32)
                n147 = local read "DetCntr"() -> (w305:tag)
                n148 = local read "LS_APD_Dl_us"() -> (w293:dbl)
                n149 = local read "APDTime_us"() -> (w291:dbl)
                n150 = local read "PulseCount"() -> (w299:i32)
                n151 = local read "LaserTime_us"() -> (w335:dbl)
                n152 = local read "LaserCntr"() -> (w348:tag)
                n153 = local read "MWCntr"() -> (w337:tag)
                n154 = expression code="1E-6*x"(w294) -> (w274:dbl)
                n155 = expression code="1E-6*x"(w298) -> (w297:dbl)
                n156 = expression code="1E-6*x"(w296) -> (w295:dbl)
                n157 = local read "APDCntr"() -> (w333:tag)
                n158 = local read "APDOutput"() -> (w277:tag)
                n159 = local read "DetInput"() -> (w307:tag)
                n160 = To Double Precision Float(number=w263) -> (double precision float=w269:dbl)
                n161 = call-poly <vilib>:"DAQmx Create Virtual Channel.vi"("edge"=w310, "counter"=w305, "name to assign"="DetCntTask1", "error in"=w308) -> ("task out"=w309:refnum<k21>, "error out"=w306:errorcluster)  [unwired: 10 in]
                n162 = call-poly <vilib>:"DAQmx Create Virtual Channel.vi"("high time"=w295, "low time"=w297, "counter"=w337, "name to assign"="MWTask1", "error in"=w308, "idle state"=w334, "initial delay"="Mw initial delay(s)") -> ("task out"=w344:refnum<k21>, "error out"=w343:errorcluster)  [unwired: 7 in]
                n163 = expression code="1E-6*x"(w293) -> (w292:dbl)
                n164 = expression code="1E-6*x"(w291) -> (w290:dbl)
                n165 = expression code="1E-6*x"(w335) -> (w300:dbl)
                n166 = Compound Arithmetic op=ADD(w297, w295) -> (w272:dbl)
                n167 = Multiply(x=w269, y=w272) -> (x*y=w271:dbl)
                n168 = Compound Arithmetic op=ADD(w274, w271) -> (w273:dbl)
                n169 = property class="DAQmx - Voie"(reference=w309, error in=w306, "CI.ComptFronts.Term"=w307) -> (reference out=w281:refnum<k21>, error out=w279:errorcluster)
                n170 = Compound Arithmetic op=ADD(w273, w292) -> (w268:dbl)
                n171 = call-poly <vilib>:"DAQmx Create Virtual Channel.vi"("high time"=w290, "low time"=w268, "counter"=w333, "name to assign"="APDTask1", "error in"=w308, "idle state"=w332, "initial delay"=w268) -> ("task out"=w313:refnum<k21>, "error out"=w312:errorcluster)  [unwired: 7 in]
                n172 = local read "Laser In/Out"() -> (w322:tag)
                n173 = local read "MW In/Out"() -> (w311:tag)
                n174 = call-poly <vilib>:"DAQmx Create Virtual Channel.vi"("high time"=w300, "low time"=w273, "counter"=w348, "name to assign"="LaserTask1", "error in"=w308, "idle state"=w347, "initial delay"=5e-05) -> ("task out"=w284:refnum<k21>, "error out"=w351:errorcluster)  [unwired: 7 in]
                n175 = Add(x=w300, y=w273) -> (x+y=w259:dbl)
                n176 = property class="DAQmx - Voie"(reference=w344, error in=w343, "CO.Pulse.Term"=w311) -> (reference out=w341:refnum<k21>, error out=w342:errorcluster)
                n177 = property class="DAQmx - Voie"(reference=w313, error in=w312, "CO.Pulse.Term"=w277) -> (reference out=w328:refnum<k21>, error out=w329:errorcluster)
                n178 = To Double Precision Float(number=w299) -> (double precision float=w287:dbl)
                n179 = property class="DAQmx - Voie"(reference=w284, error in=w351, "CO.Pulse.Term"=w322) -> (reference out=w349:refnum<k21>, error out=w350:errorcluster)
                n180 = call-poly <vilib>:"DAQmx Timing.vi"("task/channels in"=w341, "sample mode"=w336, "samples per channel"=w263, "error in"=w342) -> ("task out"=w339:refnum<k21>, "error out"=w338:errorcluster)  [unwired: 10 in]
                n181 = Multiply(x=w287, y=w259) -> (x*y=w288:dbl)
                n182 = call-poly <vilib>:"DAQmx Timing.vi"("task/channels in"=w328, "sample mode"=w323, "samples per channel"=1, "error in"=w329) -> ("task out"=w326:refnum<k21>, "error out"=w325:errorcluster)  [unwired: 10 in]
                n183 = property class="DAQmx - Déclenchement"(reference=w281, error in=w279, "Pause.TypeDécl"=w280, "Pause.NivNum.Src"=w277, "Pause.NivNum.Quand"=w276) -> (reference out=w264:refnum<k21>, error out=w278:errorcluster)
                n184 = call-poly <vilib>:"DAQmx Timing.vi"("task/channels in"=w349, "sample mode"=w352, "samples per channel"=w299, "error in"=w350) -> ("task out"=w267:refnum<k21>, "error out"=w302:errorcluster)  [unwired: 10 in]
                n185 = call-poly <vilib>:"DAQmx Trigger.vi"("task/channels in"=w339, "source"=w322, "edge"=w289, "error in"=w338) -> ("task out"=w345:refnum<k21>, "error out"=w346:errorcluster)  [unwired: 10 in]
                n186 = call-poly <vilib>:"DAQmx Trigger.vi"("task/channels in"=w326, "source"=w322, "edge"=w289, "error in"=w325) -> ("task out"=w330:refnum<k21>, "error out"=w331:errorcluster)  [unwired: 10 in]
                n187 = local write "AcqTime"(w288) -> ()
                n188 = expression code="1E6*x"(w259) -> (w258:dbl)
                n189 = property class="DAQmx - Déclenchement"(reference=w345, error in=w346, "Start.Retriggerable"=TRUE ("Démarr.Redéclenchable")) -> (reference out=w266:refnum<k21>, error out=w304:errorcluster)
                n190 = local write "MWTask"(w266) -> ()
                n191 = property class="DAQmx - Déclenchement"(reference=w330, error in=w331, "Start.Retriggerable"=TRUE ("Démarr.Redéclenchable")) -> (reference out=w265:refnum<k21>, error out=w303:errorcluster)
                n192 = local write "APDTask"(w265) -> ()
                n193 = local write "LaserTask"(w267) -> ()
                n194 = local write "Period(us)"(w258) -> ()
                n195 = Merge Errors(w302, w304, w303, w278) -> (w301:errorcluster)
                n196 = Bundle By Name(cluster=w260, "Functions"=DAQ6363_Func."PulsedODMR (Pulses)") -> (w262:refnum<class "DAQ6363.lvclass">)
                n197 = Array Size(array=w316) -> (size(s)=w319:i32)
                n198 = local write "DetCntTask"(w264) -> ()
                n199 = Initialize Array(TRUE, w319) -> (w317:bool[])
                n200 = property class="DAQ6363.lvclass"(reference=w262, error in=w301, "Accessor:SubDatDisplayNm"=w320, "Accessor:SubScanTable(y)"=dbl[] [] ("SubScanTable(y)"), "Accessor:ArrayDatNm"=w320, "Accessor:DataNames"=w316, "Accessor:SubVarParNm X"=w320, "Accessor:SubVarParNm Y"=w320, "Accessor:DatDisplayNm"=w320, "Accessor:ShowInstrNm"=w317) -> (reference out=w314:refnum<class "DAQ6363.lvclass">, error out=w315:errorcluster)
              }
              frame "Pulsed ODMR AWG" {
                w370 = 10214 items=["Haut"=10192, "Bas"=10214] ("Pause.NivNum.Quand")
                w374 = 10152 items=["Niveau analogique"=10101, "Fenêtre analogique"=10103, "Niveau numérique"=10152, "Pattern numérique"=10398, "Aucun"=10230] ("Pause.TypeDécl")
                w396 = 10280 items=["Montant"=10280, "Descendant"=10171] ("edge")
                w405 = string[] [] ("SubDatDisplayNm")
                w401 = string[] ["PulsedCounts(Cnt)"]
                w408 = 10178 items=["Échantillons finis"=10178, "Échantillons continus"=10123, "Point par point avec cadencement matériel"=12522] ("sample mode")
                w417 = 10214 items=["Haut"=10192, "Bas"=10214] ("idle state")
                n201 = local read "PulseCount"() -> (w388:i32)
                n202 = local read "LaserTime_us"() -> (w419:dbl)
                n203 = local read "LS_MW_Dl_us"() -> (w387:dbl)
                n204 = local read "MWTime_us"() -> (w385:dbl)
                n205 = local read "MW_LS_Dl_us"() -> (w383:dbl)
                n206 = local read "DetCntr"() -> (w392:tag)
                n207 = local read "LS_APD_Dl_us"() -> (w382:dbl)
                n208 = local read "MWP"() -> (w364:i32)
                n209 = local read "APDTime_us"() -> (w381:dbl)
                n210 = expression code="1E-6*x"(w383) -> (w369:dbl)
                n211 = local read "APDCntr"() -> (w418:tag)
                n212 = expression code="1E-6*x"(w387) -> (w386:dbl)
                n213 = expression code="1E-6*x"(w385) -> (w384:dbl)
                n214 = local read "APDOutput"() -> (w371:tag)
                n215 = local read "DetInput"() -> (w394:tag)
                n216 = To Double Precision Float(number=w364) -> (double precision float=w359:dbl)
                n217 = call-poly <vilib>:"DAQmx Create Virtual Channel.vi"("edge"=w396, "counter"=w392, "name to assign"="DetCntTask1", "error in"=w360) -> ("task out"=w395:refnum<k21>, "error out"=w393:errorcluster)  [unwired: 10 in]
                n218 = expression code="1E-6*x"(w419) -> (w389:dbl)
                n219 = expression code="1E-6*x"(w382) -> (w357:dbl)
                n220 = expression code="1E-6*x"(w381) -> (w380:dbl)
                n221 = Compound Arithmetic op=ADD(w386, w384) -> (w358:dbl)
                n222 = Multiply(x=w358, y=w359) -> (x*y=w367:dbl)
                n223 = property class="DAQmx - Voie"(reference=w395, error in=w393, "CI.ComptFronts.Term"=w394) -> (reference out=w375:refnum<k21>, error out=w373:errorcluster)
                n224 = call-poly <vilib>:"DAQmx Create Virtual Channel.vi"("high time"=w380, "low time"=w357, "counter"=w418, "name to assign"="APDTask1", "error in"=w360, "idle state"=w417) -> ("task out"=w398:refnum<k21>, "error out"=w397:errorcluster)  [unwired: 8 in]
                n225 = local read "Laser In/Out"() -> (w407:tag)
                n226 = Compound Arithmetic op=ADD(w369, w367) -> (w368:dbl)
                n227 = local read "APDGateEdge"() -> (w353:i32)
                n228 = Add(x=w389, y=w368) -> (x+y=w356:dbl)
                n229 = property class="DAQmx - Voie"(reference=w398, error in=w397, "CO.Pulse.Term"=w371, "CO.ActiverAttenteIniAuRedéclenchement"=TRUE) -> (reference out=w413:refnum<k21>, error out=w414:errorcluster)
                n230 = To Double Precision Float(number=w388) -> (double precision float=w378:dbl)
                n231 = Multiply(x=w378, y=w356) -> (x*y=w379:dbl)
                n232 = call-poly <vilib>:"DAQmx Timing.vi"("task/channels in"=w413, "sample mode"=w408, "samples per channel"=1, "error in"=w414) -> ("task out"=w411:refnum<k21>, "error out"=w410:errorcluster)  [unwired: 10 in]
                n233 = expression code="1E6*x"(w356) -> (w355:dbl)
                n234 = property class="DAQmx - Déclenchement"(reference=w375, error in=w373, "Pause.TypeDécl"=w374, "Pause.NivNum.Src"=w371, "Pause.NivNum.Quand"=w370) -> (reference out=w365:refnum<k21>, error out=w372:errorcluster)
                n235 = call-poly <vilib>:"DAQmx Trigger.vi"("task/channels in"=w411, "source"=w407, "edge"=w353, "error in"=w410) -> ("task out"=w415:refnum<k21>, "error out"=w416:errorcluster)  [unwired: 10 in]
                n236 = local write "AcqTime"(w379) -> ()
                n237 = local write "Period(us)"(w355) -> ()
                n238 = property class="DAQmx - Déclenchement"(reference=w415, error in=w416, "Start.Retriggerable"=TRUE ("Démarr.Redéclenchable")) -> (reference out=w366:refnum<k21>, error out=w391:errorcluster)
                n239 = Merge Errors(w391, w372) -> (w390:errorcluster)
                n240 = local write "APDTask"(w366) -> ()
                n241 = local write "DetCntTask"(w365) -> ()
                n242 = Bundle By Name(cluster=w361, "Functions"=DAQ6363_Func."PulsedODMR_AWG (Pulses)") -> (w363:refnum<class "DAQ6363.lvclass">)
                n243 = Array Size(array=w401) -> (size(s)=w404:i32)
                n244 = Initialize Array(TRUE, w404) -> (w402:bool[])
                n245 = property class="DAQ6363.lvclass"(reference=w363, error in=w390, "Accessor:SubDatDisplayNm"=w405, "Accessor:SubScanTable(y)"=dbl[] [] ("SubScanTable(y)"), "Accessor:ArrayDatNm"=w405, "Accessor:DataNames"=w401, "Accessor:SubVarParNm X"=w405, "Accessor:SubVarParNm Y"=w405, "Accessor:DatDisplayNm"=w405, "Accessor:ShowInstrNm"=w402) -> (reference out=w399:refnum<class "DAQ6363.lvclass">, error out=w400:errorcluster)
              }
              frame "Diff Pulsed ODMR AWG" {
                w421 = string[] ["PulsedCountsOn(Cnt)", "PulsedCountsOff(Cnt)", "PulsedCountDiff(Cnt)"]
                w438 = 10214 items=["Haut"=10192, "Bas"=10214] ("Pause.NivNum.Quand")
                w442 = 10152 items=["Niveau analogique"=10101, "Fenêtre analogique"=10103, "Niveau numérique"=10152, "Pattern numérique"=10398, "Aucun"=10230] ("Pause.TypeDécl")
                w464 = 10280 items=["Montant"=10280, "Descendant"=10171] ("edge")
                w472 = string[] [] ("SubDatDisplayNm")
                w475 = 10178 items=["Échantillons finis"=10178, "Échantillons continus"=10123, "Point par point avec cadencement matériel"=12522] ("sample mode")
                w484 = 10214 items=["Haut"=10192, "Bas"=10214] ("idle state")
                n246 = local read "LS_MW_Dl_us"() -> (w455:dbl)
                n247 = local read "MWTime_us"() -> (w453:dbl)
                n248 = local read "MW_LS_Dl_us"() -> (w451:dbl)
                n249 = local read "PulseCount"() -> (w456:i32)
                n250 = local read "LaserTime_us"() -> (w486:dbl)
                n251 = local read "MWP"() -> (w432:i32)
                n252 = local read "DetCntr"() -> (w460:tag)
                n253 = local read "LS_APD_Dl_us"() -> (w450:dbl)
                n254 = local read "APDTime_us"() -> (w449:dbl)
                n255 = expression code="1E-6*x"(w451) -> (w437:dbl)
                n256 = expression code="1E-6*x"(w455) -> (w454:dbl)
                n257 = expression code="1E-6*x"(w453) -> (w452:dbl)
                n258 = local read "APDCntr"() -> (w485:tag)
                n259 = local read "APDOutput"() -> (w439:tag)
                n260 = To Double Precision Float(number=w432) -> (double precision float=w427:dbl)
                n261 = local read "DetInput"() -> (w462:tag)
                n262 = call-poly <vilib>:"DAQmx Create Virtual Channel.vi"("edge"=w464, "counter"=w460, "name to assign"="DetCntTask1", "error in"=w428) -> ("task out"=w463:refnum<k21>, "error out"=w461:errorcluster)  [unwired: 10 in]
                n263 = expression code="1E-6*x"(w486) -> (w457:dbl)
                n264 = expression code="1E-6*x"(w450) -> (w425:dbl)
                n265 = expression code="1E-6*x"(w449) -> (w448:dbl)
                n266 = Compound Arithmetic op=ADD(w454, w452) -> (w426:dbl)
                n267 = Multiply(x=w426, y=w427) -> (x*y=w435:dbl)
                n268 = Compound Arithmetic op=ADD(w437, w435) -> (w436:dbl)
                n269 = property class="DAQmx - Voie"(reference=w463, error in=w461, "CI.ComptFronts.Term"=w462) -> (reference out=w443:refnum<k21>, error out=w441:errorcluster)
                n270 = call-poly <vilib>:"DAQmx Create Virtual Channel.vi"("high time"=w448, "low time"=w425, "counter"=w485, "name to assign"="APDTask1", "error in"=w428, "idle state"=w484) -> ("task out"=w466:refnum<k21>, "error out"=w465:errorcluster)  [unwired: 8 in]
                n271 = local read "Laser In/Out"() -> (w474:tag)
                n272 = local read "APDGateEdge"() -> (w420:i32)
                n273 = Add(x=w457, y=w436) -> (x+y=w424:dbl)
                n274 = property class="DAQmx - Voie"(reference=w466, error in=w465, "CO.Pulse.Term"=w439, "CO.ActiverAttenteIniAuRedéclenchement"=TRUE) -> (reference out=w480:refnum<k21>, error out=w481:errorcluster)
                n275 = To Double Precision Float(number=w456) -> (double precision float=w446:dbl)
                n276 = Multiply(x=w446, y=w424) -> (x*y=w447:dbl)
                n277 = call-poly <vilib>:"DAQmx Timing.vi"("task/channels in"=w480, "sample mode"=w475, "samples per channel"=1, "error in"=w481) -> ("task out"=w478:refnum<k21>, "error out"=w477:errorcluster)  [unwired: 10 in]
                n278 = expression code="1E6*x"(w424) -> (w423:dbl)
                n279 = property class="DAQmx - Déclenchement"(reference=w443, error in=w441, "Pause.TypeDécl"=w442, "Pause.NivNum.Src"=w439, "Pause.NivNum.Quand"=w438) -> (reference out=w433:refnum<k21>, error out=w440:errorcluster)
                n280 = call-poly <vilib>:"DAQmx Trigger.vi"("task/channels in"=w478, "source"=w474, "edge"=w420, "error in"=w477) -> ("task out"=w482:refnum<k21>, "error out"=w483:errorcluster)  [unwired: 10 in]
                n281 = local write "AcqTime"(w447) -> ()
                n282 = local write "Period(us)"(w423) -> ()
                n283 = property class="DAQmx - Déclenchement"(reference=w482, error in=w483, "Start.Retriggerable"=TRUE ("Démarr.Redéclenchable")) -> (reference out=w434:refnum<k21>, error out=w459:errorcluster)
                n284 = Merge Errors(w459, w440) -> (w458:errorcluster)
                n285 = local write "APDTask"(w434) -> ()
                n286 = local write "DetCntTask"(w433) -> ()
                n287 = Bundle By Name(cluster=w429, "Functions"=DAQ6363_Func."DiffPulsedODMR_AWG (Pulses)") -> (w431:refnum<class "DAQ6363.lvclass">)
                n288 = Array Size(array=w421) -> (size(s)=w471:i32)
                n289 = Initialize Array(TRUE, w471) -> (w469:bool[])
                n290 = property class="DAQ6363.lvclass"(reference=w431, error in=w458, "Accessor:SubDatDisplayNm"=w472, "Accessor:SubScanTable(y)"=dbl[] [] ("SubScanTable(y)"), "Accessor:ArrayDatNm"=w472, "Accessor:DataNames"=w421, "Accessor:SubVarParNm X"=w472, "Accessor:SubVarParNm Y"=w472, "Accessor:DatDisplayNm"=w472, "Accessor:ShowInstrNm"=w469) -> (reference out=w467:refnum<class "DAQ6363.lvclass">, error out=w468:errorcluster)
              }
              frame "Diff ODMR Sgl Pulse AWG" {
                w500 = 10214 items=["Haut"=10192, "Bas"=10214] ("Pause.NivNum.Quand")
                w505 = 10280 items=["Montant"=10280, "Descendant"=10171] ("edge")
                w519 = 10178 items=["Échantillons finis"=10178, "Échantillons continus"=10123, "Point par point avec cadencement matériel"=12522] ("sample mode")
                w525 = 10214 items=["Haut"=10192, "Bas"=10214] ("idle state")
                w531 = string[] ["PulsedCountsOn(Cnt)", "PulsedCountsOff(Cnt)", "PulsedCountDiff(Cnt)"]
                w544 = 10214 items=["Haut"=10192, "Bas"=10214] ("Pause.NivNum.Quand")
                w494 = 10152 items=["Niveau analogique"=10101, "Fenêtre analogique"=10103, "Niveau numérique"=10152, "Pattern numérique"=10398, "Aucun"=10230] ("Pause.TypeDécl")
                w566 = 10280 items=["Montant"=10280, "Descendant"=10171] ("edge")
                w574 = string[] [] ("SubDatDisplayNm")
                w576 = 10178 items=["Échantillons finis"=10178, "Échantillons continus"=10123, "Point par point avec cadencement matériel"=12522] ("sample mode")
                w585 = 10214 items=["Haut"=10192, "Bas"=10214] ("idle state")
                n291 = local read "LS_APD_Dl_us 2"() -> (w517:dbl)
                n292 = local read "APDOutput"() -> (w499:tag)
                n293 = local read "DetCntr 2"() -> (w506:tag)
                n294 = local read "LS_APD_Dl_us"() -> (w552:dbl)
                n295 = local read "APDTime_us"() -> (w551:dbl)
                n296 = local read "MWP"() -> (w538:i32)
                n297 = local read "LS_MW_Dl_us"() -> (w557:dbl)
                n298 = local read "MWTime_us"() -> (w555:dbl)
                n299 = local read "PulseCount"() -> (w558:i32)
                n300 = local read "LaserTime_us"() -> (w587:dbl)
                n301 = local read "MW_LS_Dl_us"() -> (w553:dbl)
                n302 = local read "DetCntr"() -> (w562:tag)
                n303 = local read "APDGateCntr2"() -> (w526:tag)
                n304 = local read "APDCntr"() -> (w586:tag)
                n305 = expression code="1E-6*x"(w553) -> (w543:dbl)
                n306 = To Double Precision Float(number=w538) -> (double precision float=w530:dbl)
                n307 = expression code="1E-6*x"(w557) -> (w556:dbl)
                n308 = expression code="1E-6*x"(w555) -> (w554:dbl)
                n309 = local read "DetInput"() -> (w564:tag)
                n310 = expression code="1E-6*x"(0.05 ("low time")) -> (w487:dbl)
                n311 = expression code="1E-6*x"(w552) -> (w490:dbl)
                n312 = expression code="1E-6*x"(w551) -> (w528:dbl)
                n313 = call-poly <vilib>:"DAQmx Create Virtual Channel.vi"("edge"=w566, "counter"=w562, "name to assign"="DetCntTask1", "error in"=w504) -> ("task out"=w565:refnum<k21>, "error out"=w563:errorcluster)  [unwired: 10 in]
                n314 = expression code="1E-6*x"(w587) -> (w559:dbl)
                n315 = expression code="1E-6*x"(w517) -> (w489:dbl)
                n316 = call-poly <vilib>:"DAQmx Create Virtual Channel.vi"("edge"=w505, "counter"=w506, "name to assign"="DetCntTask2", "error in"=w504) -> ("task out"=w501:refnum<k21>, "error out"=w503:errorcluster)  [unwired: 10 in]
                n317 = Compound Arithmetic op=ADD(w556, w554) -> (w529:dbl)
                n318 = call-poly <vilib>:"DAQmx Create Virtual Channel.vi"("high time"=w528, "low time"=w487, "counter"=w526, "name to assign"="APDTask2", "error in"=w504, "idle state"=w525, "initial delay"=w489) -> ("task out"=w522:refnum<k21>, "error out"=w523:errorcluster)  [unwired: 7 in]
                n319 = local read "APDOutput 2"() -> (w498:tag)
                n320 = Multiply(x=w530, y=w529) -> (x*y=w541:dbl)
                n321 = property class="DAQmx - Voie"(reference=w565, error in=w563, "CI.ComptFronts.Term"=w564) -> (reference out=w546:refnum<k21>, error out=w545:errorcluster)
                n322 = local read "MW In/Out"() -> (w491:tag)
                n323 = call-poly <vilib>:"DAQmx Create Virtual Channel.vi"("high time"=w528, "low time"=w487, "counter"=w586, "name to assign"="APDTask1", "error in"=w504, "idle state"=w585, "initial delay"=w490) -> ("task out"=w568:refnum<k21>, "error out"=w567:errorcluster)  [unwired: 7 in]
                n324 = local read "DetInput2"() -> (w502:tag)
                n325 = local read "APDGateEdge"() -> (w515:i32)
                n326 = Compound Arithmetic op=ADD(w543, w541) -> (w542:dbl)
                n327 = local read "Laser In/Out"() -> (w516:tag)
                n328 = Add(x=w559, y=w542) -> (x+y=w534:dbl)
                n329 = property class="DAQmx - Voie"(reference=w501, error in=w503, "CI.ComptFronts.Term"=w502) -> (reference out=w497:refnum<k21>, error out=w496:errorcluster)
                n330 = property class="DAQmx - Voie"(reference=w568, error in=w567, "CO.Pulse.Term"=w499, "CO.ActiverAttenteIniAuRedéclenchement"=TRUE) -> (reference out=w581:refnum<k21>, error out=w582:errorcluster)
                n331 = property class="DAQmx - Voie"(reference=w522, error in=w523, "CO.Pulse.Term"=w498, "CO.ActiverAttenteIniAuRedéclenchement"=TRUE) -> (reference out=w521:refnum<k21>, error out=w520:errorcluster)
                n332 = To Double Precision Float(number=w558) -> (double precision float=w549:dbl)
                n333 = Multiply(x=w549, y=w534) -> (x*y=w550:dbl)
                n334 = call-poly <vilib>:"DAQmx Timing.vi"("task/channels in"=w581, "sample mode"=w576, "samples per channel"=1, "error in"=w582) -> ("task out"=w579:refnum<k21>, "error out"=w578:errorcluster)  [unwired: 10 in]
                n335 = expression code="1E6*x"(w534) -> (w533:dbl)
                n336 = call-poly <vilib>:"DAQmx Timing.vi"("task/channels in"=w521, "sample mode"=w519, "samples per channel"=1, "error in"=w520) -> ("task out"=w514:refnum<k21>, "error out"=w510:errorcluster)  [unwired: 10 in]
                n337 = property class="DAQmx - Déclenchement"(reference=w546, error in=w545, "Pause.TypeDécl"=w494, "Pause.NivNum.Src"=w499, "Pause.NivNum.Quand"=w544) -> (reference out=w539:refnum<k21>, error out=w493:errorcluster)
                n338 = call-poly <vilib>:"DAQmx Trigger.vi"("task/channels in"=w579, "source"=w516, "edge"=w515, "error in"=w578) -> ("task out"=w583:refnum<k21>, "error out"=w584:errorcluster)  [unwired: 10 in]
                n339 = property class="DAQmx - Déclenchement"(reference=w497, error in=w496, "Pause.TypeDécl"=w494, "Pause.NivNum.Src"=w498, "Pause.NivNum.Quand"=w500) -> (reference out=w495:refnum<k21>, error out=w492:errorcluster)
                n340 = local write "AcqTime"(w550) -> ()
                n341 = local write "Period(us)"(w533) -> ()
                n342 = call-poly <vilib>:"DAQmx Trigger.vi"("task/channels in"=w514, "source"=w491, "edge"=w515, "error in"=w510) -> ("task out"=w512:refnum<k21>, "error out"=w511:errorcluster)  [unwired: 10 in]
                n343 = property class="DAQmx - Déclenchement"(reference=w583, error in=w584, "Start.Retriggerable"=TRUE ("Démarr.Redéclenchable")) -> (reference out=w540:refnum<k21>, error out=w561:errorcluster)
                n344 = property class="DAQmx - Déclenchement"(reference=w512, error in=w511, "Start.Retriggerable"=TRUE ("Démarr.Redéclenchable")) -> (reference out=w508:refnum<k21>, error out=w509:errorcluster)
                n345 = Merge Errors(w561, w509, w492, w493) -> (w560:errorcluster)
                n346 = local write "APDTask"(w540) -> ()
                n347 = local write "DetCntTask"(w539) -> ()
                n348 = local write "APD2GateTask"(w508) -> ()
                n349 = Bundle By Name(cluster=w535, "Functions"=DAQ6363_Func."DiffODMRSglPulseAWG (Pulses)") -> (w537:refnum<class "DAQ6363.lvclass">)
                n350 = Array Size(array=w531) -> (size(s)=w573:i32)
                n351 = Initialize Array(TRUE, w573) -> (w571:bool[])
                n352 = local write "Det2CntTask"(w495) -> ()
                n353 = property class="DAQ6363.lvclass"(reference=w537, error in=w560, "Accessor:SubDatDisplayNm"=w574, "Accessor:SubScanTable(y)"=dbl[] [] ("SubScanTable(y)"), "Accessor:ArrayDatNm"=w574, "Accessor:DataNames"=w531, "Accessor:SubVarParNm X"=w574, "Accessor:SubVarParNm Y"=w574, "Accessor:DatDisplayNm"=w574, "Accessor:ShowInstrNm"=w571) -> (reference out=w569:refnum<class "DAQ6363.lvclass">, error out=w570:errorcluster)
              }
              frame "Gated Pulse Count" {
                w593 = string[] ["PulsedCountsCh1(Cnt)", "PulsedCountsCh2(Cnt)", "PulsedCountsSum(Cnt)"]
                w602 = string[] [] ("SubDatDisplayNm")
                n354 = local read "Channel 2"() -> (w591:bool)
                n355 = case shown="Faux" w591 {
                  selector: w591 -> [_ w610]
                  tunnel: w592 -> [w608 w611]
                  tunnel: [w608 w609] -> w590
                  frame False {
                  }
                  frame True {
                    n356 = property on="Channel 1" class="Bool (strict)"(error in=w611, "Val(Sgnl)"=w610) -> (error out=w609:errorcluster)  [unwired: 1 in, 1 out]
                  }
                }
                n357 = local read "Channel 1"() -> (w588:bool)
                n358 = case shown="Faux" w588 {
                  selector: w588 -> [_ w605]
                  tunnel: w590 -> [w604 w607]
                  tunnel: [w604 w606] -> w589
                  frame False {
                  }
                  frame True {
                    n359 = property on="Channel 1" class="Bool (strict)"(error in=w607, "Val(Sgnl)"=w605) -> (error out=w606:errorcluster)  [unwired: 1 in, 1 out]
                  }
                }
                n360 = Bundle By Name(cluster=w594, "Functions"=DAQ6363_Func."DiffODMRSglPulseAWG (Pulses)") -> (w596:refnum<class "DAQ6363.lvclass">)
                n361 = Array Size(array=w593) -> (size(s)=w601:i32)
                n362 = Initialize Array(TRUE, w601) -> (w599:bool[])
                n363 = property class="DAQ6363.lvclass"(reference=w596, error in=w589, "Accessor:SubDatDisplayNm"=w602, "Accessor:SubScanTable(y)"=dbl[] [] ("SubScanTable(y)"), "Accessor:ArrayDatNm"=w602, "Accessor:DataNames"=w593, "Accessor:SubVarParNm X"=w602, "Accessor:SubVarParNm Y"=w602, "Accessor:DatDisplayNm"=w602, "Accessor:ShowInstrNm"=w599) -> (reference out=w597:refnum<class "DAQ6363.lvclass">, error out=w598:errorcluster)
              }
              frame "Diff Pulsed ODMR" {
                w618 = string[] ["PulsedCountsOn(Cnt)", "PulsedCountsOff(Cnt)", "PulsedCountsDiff(Cnt)"]
                w631 = 10214 items=["Haut"=10192, "Bas"=10214] ("Pause.NivNum.Quand")
                w635 = 10152 items=["Niveau analogique"=10101, "Fenêtre analogique"=10103, "Niveau numérique"=10152, "Pattern numérique"=10398, "Aucun"=10230] ("Pause.TypeDécl")
                w644 = 10171 items=["Montant"=10280, "Descendant"=10171] ("edge")
                w665 = 10280 items=["Montant"=10280, "Descendant"=10171] ("edge")
                w674 = string[] [] ("SubDatDisplayNm")
                w677 = 10178 items=["Échantillons finis"=10178, "Échantillons continus"=10123, "Point par point avec cadencement matériel"=12522] ("sample mode")
                w686 = 10214 items=["Haut"=10192, "Bas"=10214] ("idle state")
                w688 = 10214 items=["Haut"=10192, "Bas"=10214] ("idle state")
                w690 = 10178 items=["Échantillons finis"=10178, "Échantillons continus"=10123, "Point par point avec cadencement matériel"=12522] ("sample mode")
                w701 = 10192 items=["Haut"=10192, "Bas"=10214] ("idle state")
                w706 = 10178 items=["Échantillons finis"=10178, "Échantillons continus"=10123, "Point par point avec cadencement matériel"=12522]  # Mode d'échantillonnage
                n364 = local read "PulseCount"() -> (w654:i32)
                n365 = local read "LaserTime_us"() -> (w689:dbl)
                n366 = local read "LaserCntr"() -> (w702:tag)
                n367 = local read "LS_MW_Dl_us"() -> (w653:dbl)
                n368 = local read "MWTime_us"() -> (w651:dbl)
                n369 = local read "MW_LS_Dl_us"() -> (w649:dbl)
                n370 = local read "MWP"() -> (w617:i32)
                n371 = local read "DetCntr"() -> (w660:tag)
                n372 = local read "LS_APD_Dl_us"() -> (w648:dbl)
                n373 = local read "APDTime_us"() -> (w646:dbl)
                n374 = local read "MWCntr"() -> (w691:tag)
                n375 = expression code="1E-6*x"(w649) -> (w629:dbl)
                n376 = expression code="1E-6*x"(w653) -> (w652:dbl)
                n377 = expression code="1E-6*x"(w651) -> (w650:dbl)
                n378 = local read "APDCntr"() -> (w687:tag)
                n379 = local read "APDOutput"() -> (w632:tag)
                n380 = expression code="1E-6*x"(w689) -> (w655:dbl)
                n381 = local read "DetInput"() -> (w662:tag)
                n382 = To Double Precision Float(number=w617) -> (double precision float=w624:dbl)
                n383 = call-poly <vilib>:"DAQmx Create Virtual Channel.vi"("edge"=w665, "counter"=w660, "name to assign"="DetCntTask1", "error in"=w663) -> ("task out"=w664:refnum<k21>, "error out"=w661:errorcluster)  [unwired: 10 in]
                n384 = call-poly <vilib>:"DAQmx Create Virtual Channel.vi"("high time"=w650, "low time"=w652, "counter"=w691, "name to assign"="MWTask1", "error in"=w663, "idle state"=w688, "initial delay"="Mw initial delay(s) 2") -> ("task out"=w698:refnum<k21>, "error out"=w697:errorcluster)  [unwired: 7 in]
                n385 = expression code="1E-6*x"(w648) -> (w647:dbl)
                n386 = expression code="1E-6*x"(w646) -> (w645:dbl)
                n387 = Compound Arithmetic op=ADD(w652, w650) -> (w627:dbl)
                n388 = Multiply(x=w624, y=w627) -> (x*y=w626:dbl)
                n389 = Compound Arithmetic op=ADD(w629, w626) -> (w628:dbl)
                n390 = property class="DAQmx - Voie"(reference=w664, error in=w661, "CI.ComptFronts.Term"=w662) -> (reference out=w636:refnum<k21>, error out=w634:errorcluster)
                n391 = Compound Arithmetic op=ADD(w628, w647) -> (w623:dbl)
                n392 = call-poly <vilib>:"DAQmx Create Virtual Channel.vi"("high time"=w645, "low time"=w623, "counter"=w687, "name to assign"="APDTask1", "error in"=w663, "idle state"=w686, "initial delay"=w623) -> ("task out"=w668:refnum<k21>, "error out"=w667:errorcluster)  [unwired: 7 in]
                n393 = local read "Laser In/Out"() -> (w676:tag)
                n394 = local read "MW In/Out"() -> (w666:tag)
                n395 = call-poly <vilib>:"DAQmx Create Virtual Channel.vi"("high time"=w655, "low time"=w628, "counter"=w702, "name to assign"="LaserTask1", "error in"=w663, "idle state"=w701, "initial delay"=5e-05) -> ("task out"=w639:refnum<k21>, "error out"=w705:errorcluster)  [unwired: 7 in]
                n396 = Add(x=w655, y=w628) -> (x+y=w613:dbl)
                n397 = property class="DAQmx - Voie"(reference=w698, error in=w697, "CO.Pulse.Term"=w666) -> (reference out=w695:refnum<k21>, error out=w696:errorcluster)
                n398 = property class="DAQmx - Voie"(reference=w668, error in=w667, "CO.Pulse.Term"=w632) -> (reference out=w682:refnum<k21>, error out=w683:errorcluster)
                n399 = To Double Precision Float(number=w654) -> (double precision float=w642:dbl)
                n400 = property class="DAQmx - Voie"(reference=w639, error in=w705, "CO.Pulse.Term"=w676) -> (reference out=w703:refnum<k21>, error out=w704:errorcluster)
                n401 = call-poly <vilib>:"DAQmx Timing.vi"("task/channels in"=w695, "sample mode"=w690, "samples per channel"=w617, "error in"=w696) -> ("task out"=w693:refnum<k21>, "error out"=w692:errorcluster)  [unwired: 10 in]
                n402 = Multiply(x=w642, y=w613) -> (x*y=w643:dbl)
                n403 = call-poly <vilib>:"DAQmx Timing.vi"("task/channels in"=w682, "sample mode"=w677, "samples per channel"=1, "error in"=w683) -> ("task out"=w680:refnum<k21>, "error out"=w679:errorcluster)  [unwired: 10 in]
                n404 = expression code="1E6*x"(w613) -> (w612:dbl)
                n405 = property class="DAQmx - Déclenchement"(reference=w636, error in=w634, "Pause.TypeDécl"=w635, "Pause.NivNum.Src"=w632, "Pause.NivNum.Quand"=w631) -> (reference out=w619:refnum<k21>, error out=w633:errorcluster)
                n406 = call-poly <vilib>:"DAQmx Timing.vi"("task/channels in"=w703, "sample mode"=w706, "samples per channel"=w654, "error in"=w704) -> ("task out"=w622:refnum<k21>, "error out"=w657:errorcluster)  [unwired: 10 in]
                n407 = call-poly <vilib>:"DAQmx Trigger.vi"("task/channels in"=w693, "source"=w676, "edge"=w644, "error in"=w692) -> ("task out"=w699:refnum<k21>, "error out"=w700:errorcluster)  [unwired: 10 in]
                n408 = call-poly <vilib>:"DAQmx Trigger.vi"("task/channels in"=w680, "source"=w676, "edge"=w644, "error in"=w679) -> ("task out"=w684:refnum<k21>, "error out"=w685:errorcluster)  [unwired: 10 in]
                n409 = local write "AcqTime"(w643) -> ()
                n410 = local write "Period(us)"(w612) -> ()
                n411 = local write "LaserTask"(w622) -> ()
                n412 = property class="DAQmx - Déclenchement"(reference=w699, error in=w700, "Start.Retriggerable"=TRUE ("Démarr.Redéclenchable")) -> (reference out=w621:refnum<k21>, error out=w659:errorcluster)
                n413 = local write "MWTask"(w621) -> ()
                n414 = property class="DAQmx - Déclenchement"(reference=w684, error in=w685, "Start.Retriggerable"=TRUE ("Démarr.Redéclenchable")) -> (reference out=w620:refnum<k21>, error out=w658:errorcluster)
                n415 = local write "APDTask"(w620) -> ()
                n416 = Merge Errors(w657, w659, w658, w633) -> (w656:errorcluster)
                n417 = Bundle By Name(cluster=w614, "Functions"=DAQ6363_Func."DiffPulsedODMR (Pulses)") -> (w616:refnum<class "DAQ6363.lvclass">)
                n418 = Array Size(array=w618) -> (size(s)=w673:i32)
                n419 = local write "DetCntTask"(w619) -> ()
                n420 = Initialize Array(TRUE, w673) -> (w671:bool[])
                n421 = property class="DAQ6363.lvclass"(reference=w616, error in=w656, "Accessor:SubDatDisplayNm"=w674, "Accessor:SubScanTable(y)"=dbl[] [] ("SubScanTable(y)"), "Accessor:ArrayDatNm"=w674, "Accessor:DataNames"=w618, "Accessor:SubVarParNm X"=w674, "Accessor:SubVarParNm Y"=w674, "Accessor:DatDisplayNm"=w674, "Accessor:ShowInstrNm"=w671) -> (reference out=w669:refnum<class "DAQ6363.lvclass">, error out=w670:errorcluster)
              }
              frame "None", Default {
              }
            }
            n422 = call-dynamic "SetClassQueueMessage.vi"("ErrorIn(No Error)"=w179, "Menu déroulant"=w187, "DefaultDev.lvclass"=w185) -> ("sortie d'erreur"=w186:errorcluster, "DefaultDev.lvclass Out"=w184:refnum<class "DAQ6363.lvclass">)  [unwired: 7 in]
          }
          event "Channel 1": Value Change {
            w715 = string[] [] ("SubDatDisplayNm")
            w721 = T3 1 items=["UpdateClassData", "UpdateMainClass", "UpdateDataBind", "ReInitDevice", "Custom", "ClosePan"] ("Menu déroulant")
            n423 = event-data() -> ("NewVal"=w709:bool)  [unwired: 1 in]
            n424 = case shown="Vrai" w709 {
              tunnel: w722 -> [w728 w767]
              tunnel: [w726 w753] -> w711
              tunnel: [w731 w735] -> w710
              frame False {
                n425 = local read "Channel 2"() -> (w729:bool)
                n426 = local read "ReadCont"() -> (w730:bool)
                n427 = case shown="Vrai" w730 {
                  tunnel: w729 -> [_ w734]
                  frame False {
                  }
                  frame True {
                    n428 = local write "ReadCont"(w734) -> ()
                    n429 = local write "ReadCnts"(w734) -> ()
                  }
                }
                n430 = local read "DetCntTask"() -> (w724:refnum<k21>)
                n431 = local read "APDTask"() -> (w725:refnum<k21>)
                n432 = call <vilib>:"DAQmx Clear Task.vi"("task in"=w725, "error in"=w728) -> ("error out"=w727:errorcluster)  [unwired: 13 in]
                n433 = call <vilib>:"DAQmx Clear Task.vi"("task in"=w724, "error in"=w727) -> ("error out"=w726:errorcluster)  [unwired: 13 in]
                n434 = Select(t=string[] ["GatedCountsCh2(Cnt)"], s=w729, f=string[] []) -> (s? t:f=w731:string[])
              }
              frame True {
                w747 = 10214 items=["Haut"=10192, "Bas"=10214] ("Pause.NivNum.Quand")
                w744 = 10152 items=["Niveau analogique"=10101, "Fenêtre analogique"=10103, "Niveau numérique"=10152, "Pattern numérique"=10398, "Aucun"=10230] ("Pause.TypeDécl")
                w758 = 10280 items=["Montant"=10280, "Descendant"=10171] ("edge")
                w761 = 10178 items=["Échantillons finis"=10178, "Échantillons continus"=10123, "Point par point avec cadencement matériel"=12522] ("sample mode")
                w765 = 10214 items=["Haut"=10192, "Bas"=10214] ("idle state")
                n435 = local read "APDTime_us"() -> (w752:dbl)
                n436 = local read "DetCntr"() -> (w754:tag)
                n437 = local read "APDCntr"() -> (w766:tag)
                n438 = local read "APDOutput"() -> (w741:tag)
                n439 = local read "DetInput"() -> (w756:tag)
                n440 = expression code="1E-6*x"(w752) -> (w739:dbl)
                n441 = call-poly <vilib>:"DAQmx Create Virtual Channel.vi"("edge"=w758, "counter"=w754, "name to assign"="DetCntTask1", "error in"=w767) -> ("task out"=w757:refnum<k21>, "error out"=w755:errorcluster)  [unwired: 10 in]
                n442 = call-poly <vilib>:"DAQmx Create Virtual Channel.vi"("high time"=w739, "counter"=w766, "name to assign"="APDTask1", "error in"=w767, "idle state"=w765) -> ("task out"=w760:refnum<k21>, "error out"=w759:errorcluster)  [unwired: 9 in]
                n443 = expression code="1E6*x"(w739) -> (w745:dbl)
                n444 = property class="DAQmx - Voie"(reference=w757, error in=w755, "CI.ComptFronts.Term"=w756) -> (reference out=w749:refnum<k21>, error out=w748:errorcluster)
                n445 = local read "Channel 2"() -> (w736:bool)
                n446 = local write "AcqTime"(w739) -> ()
                n447 = local write "Period(us)"(w745) -> ()
                n448 = property class="DAQmx - Voie"(reference=w760, error in=w759, "CO.Pulse.Term"=w741) -> (reference out=w763:refnum<k21>, error out=w764:errorcluster)
                n449 = property class="DAQmx - Déclenchement"(reference=w749, error in=w748, "Pause.TypeDécl"=w744, "Pause.NivNum.Src"=w741, "Pause.NivNum.Quand"=w747) -> (reference out=w746:refnum<k21>, error out=w740:errorcluster)
                n450 = call-poly <vilib>:"DAQmx Timing.vi"("task/channels in"=w763, "sample mode"=w761, "samples per channel"=1, "error in"=w764) -> ("task out"=w742:refnum<k21>, "error out"=w743:errorcluster)  [unwired: 10 in]
                n451 = local write "APDTask"(w742) -> ()
                n452 = Select(t=string[] ["GatedCountsCh1(Cnt)", "GatedCountsCh2(Cnt)", "GatedCountsSum(Cnt)"], s=w736, f=string[] ["GatedCountsCh1(Cnt)"]) -> (s? t:f=w735:string[])
                n453 = local write "DetCntTask"(w746) -> ()
                n454 = Merge Errors(w743, w740) -> (w753:errorcluster)
              }
            }
            n455 = Array Size(array=w710) -> (size(s)=w714:i32)
            n456 = Initialize Array(TRUE, w714) -> (w712:bool[])
            n457 = property class="DAQ6363.lvclass"(reference=w723, error in=w711, "Accessor:SubDatDisplayNm"=w715, "Accessor:SubScanTable(y)"=dbl[] [] ("SubScanTable(y)"), "Accessor:ArrayDatNm"=w715, "Accessor:DataNames"=w710, "Accessor:SubVarParNm X"=w715, "Accessor:SubVarParNm Y"=w715, "Accessor:DatDisplayNm"=w715, "Accessor:ShowInstrNm"=w712) -> (reference out=w718:refnum<class "DAQ6363.lvclass">, error out=w720:errorcluster)
            n458 = call-dynamic "SetClassQueueMessage.vi"("ErrorIn(No Error)"=w720, "Menu déroulant"=w721, "DefaultDev.lvclass"=w718) -> ("sortie d'erreur"=w719:errorcluster, "DefaultDev.lvclass Out"=w717:refnum<class "DAQ6363.lvclass">)  [unwired: 7 in]
          }
          event "Channel 2": Value Change {
            w774 = string[] [] ("SubDatDisplayNm")
            w780 = T3 1 items=["UpdateClassData", "UpdateMainClass", "UpdateDataBind", "ReInitDevice", "Custom", "ClosePan"] ("Menu déroulant")
            n459 = event-data() -> ("NewVal"=w768:bool)  [unwired: 1 in]
            n460 = case shown="Faux" w768 {
              tunnel: w781 -> [w787 w826]
              tunnel: [w785 w812] -> w770
              tunnel: [w790 w794] -> w769
              frame False {
                n461 = local read "Channel 1"() -> (w788:bool)
                n462 = local read "ReadCont"() -> (w789:bool)
                n463 = case shown="Vrai" w789 {
                  tunnel: w788 -> [_ w793]
                  frame False {
                  }
                  frame True {
                    n464 = local write "ReadCont"(w793) -> ()
                    n465 = local write "ReadCnts"(w793) -> ()
                  }
                }
                n466 = local read "APD2GateTask"() -> (w784:refnum<k21>)
                n467 = local read "Det2CntTask"() -> (w783:refnum<k21>)
                n468 = call <vilib>:"DAQmx Clear Task.vi"("task in"=w784, "error in"=w787) -> ("error out"=w786:errorcluster)  [unwired: 13 in]
                n469 = call <vilib>:"DAQmx Clear Task.vi"("task in"=w783, "error in"=w786) -> ("error out"=w785:errorcluster)  [unwired: 13 in]
                n470 = Select(t=string[] ["GatedCountsCh1(Cnt)"], s=w788, f=string[] []) -> (s? t:f=w790:string[])
              }
              frame True {
                w806 = 10214 items=["Haut"=10192, "Bas"=10214] ("Pause.NivNum.Quand")
                w803 = 10152 items=["Niveau analogique"=10101, "Fenêtre analogique"=10103, "Niveau numérique"=10152, "Pattern numérique"=10398, "Aucun"=10230] ("Pause.TypeDécl")
                w817 = 10280 items=["Montant"=10280, "Descendant"=10171] ("edge")
                w820 = 10178 items=["Échantillons finis"=10178, "Échantillons continus"=10123, "Point par point avec cadencement matériel"=12522] ("sample mode")
                w824 = 10214 items=["Haut"=10192, "Bas"=10214] ("idle state")
                n471 = local read "APDTime_us"() -> (w811:dbl)
                n472 = local read "DetCntr 2"() -> (w813:tag)
                n473 = local read "APDGateCntr2"() -> (w825:tag)
                n474 = local read "APDOutput 2"() -> (w800:tag)
                n475 = local read "DetInput2"() -> (w815:tag)
                n476 = expression code="1E-6*x"(w811) -> (w798:dbl)
                n477 = call-poly <vilib>:"DAQmx Create Virtual Channel.vi"("edge"=w817, "counter"=w813, "name to assign"="DetCntTask1", "error in"=w826) -> ("task out"=w816:refnum<k21>, "error out"=w814:errorcluster)  [unwired: 10 in]
                n478 = call-poly <vilib>:"DAQmx Create Virtual Channel.vi"("high time"=w798, "counter"=w825, "name to assign"="APDTask1", "error in"=w826, "idle state"=w824) -> ("task out"=w819:refnum<k21>, "error out"=w818:errorcluster)  [unwired: 9 in]
                n479 = expression code="1E6*x"(w798) -> (w804:dbl)
                n480 = property class="DAQmx - Voie"(reference=w816, error in=w814, "CI.ComptFronts.Term"=w815) -> (reference out=w808:refnum<k21>, error out=w807:errorcluster)
                n481 = local read "Channel 1"() -> (w795:bool)
                n482 = local write "AcqTime"(w798) -> ()
                n483 = local write "Period(us)"(w804) -> ()
                n484 = property class="DAQmx - Voie"(reference=w819, error in=w818, "CO.Pulse.Term"=w800) -> (reference out=w822:refnum<k21>, error out=w823:errorcluster)
                n485 = property class="DAQmx - Déclenchement"(reference=w808, error in=w807, "Pause.TypeDécl"=w803, "Pause.NivNum.Src"=w800, "Pause.NivNum.Quand"=w806) -> (reference out=w805:refnum<k21>, error out=w799:errorcluster)
                n486 = call-poly <vilib>:"DAQmx Timing.vi"("task/channels in"=w822, "sample mode"=w820, "samples per channel"=1, "error in"=w823) -> ("task out"=w801:refnum<k21>, "error out"=w802:errorcluster)  [unwired: 10 in]
                n487 = local write "APD2GateTask"(w801) -> ()
                n488 = Select(t=string[] ["GatedCountsCh1(Cnt)", "GatedCountsCh2(Cnt)", "GatedCountsSum(Cnt)"], s=w795, f=string[] ["GatedCountsCh2(Cnt)"]) -> (s? t:f=w794:string[])
                n489 = local write "Det2CntTask"(w805) -> ()
                n490 = Merge Errors(w802, w799) -> (w812:errorcluster)
              }
            }
            n491 = Array Size(array=w769) -> (size(s)=w773:i32)
            n492 = Initialize Array(TRUE, w773) -> (w771:bool[])
            n493 = property class="DAQ6363.lvclass"(reference=w782, error in=w770, "Accessor:SubDatDisplayNm"=w774, "Accessor:SubScanTable(y)"=dbl[] [] ("SubScanTable(y)"), "Accessor:ArrayDatNm"=w774, "Accessor:DataNames"=w769, "Accessor:SubVarParNm X"=w774, "Accessor:SubVarParNm Y"=w774, "Accessor:DatDisplayNm"=w774, "Accessor:ShowInstrNm"=w771) -> (reference out=w777:refnum<class "DAQ6363.lvclass">, error out=w779:errorcluster)
            n494 = call-dynamic "SetClassQueueMessage.vi"("ErrorIn(No Error)"=w779, "Menu déroulant"=w780, "DefaultDev.lvclass"=w777) -> ("sortie d'erreur"=w778:errorcluster, "DefaultDev.lvclass Out"=w776:refnum<class "DAQ6363.lvclass">)  [unwired: 7 in]
          }
          event "PulseCount": Value Change {
            n495 = event-data() -> ("NewVal"=w831:i32)  [unwired: 1 in]
            n496 = local read "Pulse Function"() -> (w828:T1)
            n497 = case shown="\"Pulsed ODMR\", \"Diff Pulsed ODMR\"" w828 {
              tunnel: w831 -> [_ w837]
              tunnel: w827 -> [w832 w839]
              tunnel: [w832 w838] -> w829
              frame Default {
              }
              frame "Pulsed ODMR", "Diff Pulsed ODMR" {
                w840 = 10178 items=["Échantillons finis"=10178, "Échantillons continus"=10123, "Point par point avec cadencement matériel"=12522]  # Mode d'échantillonnage
                n498 = local read "LaserTask"() -> (w835:refnum<k21>)
                n499 = local read "Period(us)"() -> (w834:dbl)
                n500 = call-poly <vilib>:"DAQmx Timing.vi"("task/channels in"=w835, "sample mode"=w840, "samples per channel"=w837, "error in"=w839) -> ("error out"=w838:errorcluster)  [unwired: 10 in, 1 out]
                n501 = expression code="1E-6*x"(w834) -> (w833:dbl)
                n502 = Multiply(x=w837, y=w833) -> (x*y=w836:dbl)
                n503 = local write "AcqTime"(w836) -> ()
              }
            }
          }
          event "LaserLowTime": Value Change {
            n504 = event-data() -> ("NewVal"=w845:dbl)  [unwired: 1 in, 5 out]
            n505 = local read "Pulse Function"() -> (w841:T1)
            n506 = case shown="\"Pulsed ODMR\", \"Diff Pulsed ODMR\"" w841 {
              tunnel: w845 -> [_ w851]
              tunnel: w843 -> [w846 w860]
              tunnel: [w846 w853] -> w842
              frame Default {
              }
              frame "Pulsed ODMR", "Diff Pulsed ODMR" {
                w856 = 3 items=["vérifier"=2, "réserver"=4, "programmer"=3, "libérer"=5, "abandonner"=6] ("action")
                w864 = 3 items=["vérifier"=2, "réserver"=4, "programmer"=3, "libérer"=5, "abandonner"=6] ("action")
                n507 = local read "LaserTask"() -> (w861:refnum<k21>)
                n508 = local write "LaserLowTime"(w851) -> ()
                n509 = property class="DAQmx - Voie"(reference=w861, error in=w860, "CO.Impulsion.TempsBas"=w851) -> (reference out=w863:refnum<k21>, error out=w862:errorcluster)
                n510 = local read "LS_APD_Dl_us"() -> (w859:dbl)
                n511 = call <vilib>:"DAQmx Control Task.vi"("task/channels in"=w863, "action"=w864, "error in"=w862) -> ("error out"=w858:errorcluster)  [unwired: 11 in, 1 out]
                n512 = local read "APDTask"() -> (w857:refnum<k21>)
                n513 = expression code="1E-6*x"(w859) -> (w852:dbl)
                n514 = local read "LaserTime_us"() -> (w848:dbl)
                n515 = Add(x=w851, y=w852) -> (x+y=w850:dbl)
                n516 = property class="DAQmx - Voie"(reference=w857, error in=w858, "CO.Impulsion.TempsBas"=w850, "CO.Impulsion.Temps.AttenteInitiale"=w850) -> (reference out=w854:refnum<k21>, error out=w855:errorcluster)
                n517 = expression code="1E6*x"(w850) -> (w849:dbl)
                n518 = Add(x=w849, y=w848) -> (x+y=w847:dbl)
                n519 = local write "Period(us)"(w847) -> ()
                n520 = call <vilib>:"DAQmx Control Task.vi"("task/channels in"=w854, "action"=w856, "error in"=w855) -> ("error out"=w853:errorcluster)  [unwired: 11 in, 1 out]
              }
            }
          }
          event "Laser In/Out": Value Change {
            n521 = event-data() -> ("NewVal"=w869:tag)  [unwired: 1 in, 5 out]
            n522 = local read "Pulse Function"() -> (w865:T1)
            n523 = case shown="Par défaut" w865 {
              tunnel: w869 -> [_ w872]
              tunnel: w867 -> [w870 w874]
              tunnel: [w870 w873] -> w866
              frame Default {
              }
              frame "Pulsed ODMR", "Diff Pulsed ODMR" {
                n524 = local read "LaserTask"() -> (w871:refnum<k21>)
                n525 = property class="DAQmx - Voie"(reference=w871, error in=w874, "CO.Pulse.Term"=w872) -> (error out=w873:errorcluster)  [unwired: 1 out]
              }
            }
          }
          event "MW In/Out": Value Change {
            n526 = event-data() -> ("NewVal"=w879:tag)  [unwired: 1 in, 5 out]
            n527 = local read "Pulse Function"() -> (w875:T1)
            n528 = case shown="Par défaut" w875 {
              tunnel: w879 -> [_ w882]
              tunnel: w877 -> [w880 w884]
              tunnel: [w880 w883] -> w876
              frame Default {
              }
              frame "Pulsed ODMR", "Diff Pulsed ODMR" {
                n529 = local read "MWTask"() -> (w881:refnum<k21>)
                n530 = property class="DAQmx - Voie"(reference=w881, error in=w884, "CO.Pulse.Term"=w882) -> (error out=w883:errorcluster)  [unwired: 1 out]
              }
            }
          }
          event "APDOutput": Value Change {
            n531 = event-data() -> ("NewVal"=w889:tag)  [unwired: 1 in, 5 out]
            n532 = local read "Pulse Function"() -> (w885:T1)
            n533 = case shown="\"Pulsed ODMR AWG\", \"Pulsed ODMR\", \"Diff Pulsed ODMR\"" w885 {
              tunnel: w889 -> [_ w892]
              tunnel: w887 -> [w890 w894]
              tunnel: [w890 w893] -> w886
              frame Default {
              }
              frame "Pulsed ODMR AWG", "Pulsed ODMR", "Diff Pulsed ODMR" {
                n534 = local read "APDTask"() -> (w891:refnum<k21>)
                n535 = property class="DAQmx - Voie"(reference=w891, error in=w894, "CO.Pulse.Term"=w892) -> (error out=w893:errorcluster)  [unwired: 1 out]
              }
            }
          }
          event "LaserCntr", "MW_LS_Dl_us", "LS_MW_Dl_us", "MWTime_us", "LaserTime_us", "APDTime_us", "MWCntr", "APDCntr", "APDGateEdge", "LS_APD_Dl_us 2": Value Change {
            n536 = event-data() -> ("NewVal"=w899:variant)  [unwired: 1 in, 5 out]
            n537 = local read "Pulse Function"() -> (w895:T1)
            n538 = case shown="\"Diff ODMR Sgl Pulse AWG\"" w895 {
              selector: w895 -> [_ w902 w905]
              tunnel: w899 -> [_ _ _]
              tunnel: w898 -> [_ _ _]
              tunnel: w897 -> [w900 w901 w904]
              tunnel: [w900 w903 w906] -> w896
              frame "None", Default {
              }
              frame "Pulsed ODMR AWG", "Pulsed ODMR", "Diff Pulsed ODMR" {
                n539 = property on="Pulse Function" class="Énum (strict)"(error in=w901, "Val(Sgnl)"=w902) -> (error out=w903:errorcluster)  [unwired: 1 in, 1 out]
              }
              frame "Diff ODMR Sgl Pulse AWG" {
                n540 = property on="Pulse Function" class="Énum (strict)"(error in=w904, "Val(Sgnl)"=w905) -> (error out=w906:errorcluster)  [unwired: 1 in, 1 out]
              }
            }
          }
        }
        n541 = Or(x=w23, y="Stop") -> (x .or. y?=w29:bool)
      }
    }
    frame Error {
    }
  }
  "error out" <- w5
  "DAQ6363.lvclass Out" <- w3
